vi "Autonomous Independent.vi"() -> ()   [LabVIEW 2015]
doc: "This VI is called when autonomous begins, and will automatically be terminated when autonomous ends. You can carry out timed or sensor driven robot movement independently without needing to return to the caller."
uses:
  <vilib>/Rock Robotics/WPI/Relay/WPI_RelayValue.ctl
  AutonEnum.ctl
  AutonEnumGoAround.ctl
  <vilib>/Rock Robotics/WPI/Utilities/WPI_GetSetVariantRefNum.vi
  Robot Values.vi
  DriveGlobal.vi
  <vilib>/Rock Robotics/WPI/RobotDrive/WPI_RobotDriveArcadeDrive_Standard(NoSaturation).vi
  Auton1ToteEnum.ctl
panel:
  in  "turn output range 5":cluster{"output high":dbl, "output low":dbl}={"output high"=0.8, "output low"=-0.8} {"output low" format="%.2f"; "output high" format="%.2f"}
  in  "PID Turn  gains 5":T1={"proportional gain (Kc)"=0.20000000000000004, "integral time (Ti, min)"=0.0, "derivative time (Td, min)"=0.0} {"derivative time (Td, min)" format="%.3f"; "integral time (Ti, min)" format="%.3f"; "proportional gain (Kc)" format="%.3f"}
  out "Total totes 4":i32
  in  "PID Turn  gains 4":T1={"proportional gain (Kc)"=0.20000000000000004, "integral time (Ti, min)"=0.0, "derivative time (Td, min)"=0.0} {"derivative time (Td, min)" format="%.3f"; "integral time (Ti, min)" format="%.3f"; "proportional gain (Kc)" format="%.3f"}
  in  "turn output range 4":cluster{"output high":dbl, "output low":dbl}={"output high"=0.8000000000000003, "output low"=-0.8000000000000002} {"output low" format="%.2f"; "output high" format="%.2f"}
  out "Total totes 3":i32
  in  "PID Turn  gains 3":T1={"proportional gain (Kc)"=0.05, "integral time (Ti, min)"=0.01, "derivative time (Td, min)"=0.0} {"derivative time (Td, min)" format="%.3f"; "integral time (Ti, min)" format="%.3f"; "proportional gain (Kc)" format="%.3f"}
  in  "turn output range 3":cluster{"output high":dbl, "output low":dbl}={"output high"=0.4, "output low"=-0.4} {"output low" format="%.2f"; "output high" format="%.2f"}
  out "Total totes 2":i32
  in  "PID Turn  gains 2":T1={"proportional gain (Kc)"=0.05, "integral time (Ti, min)"=0.01, "derivative time (Td, min)"=0.0} {"derivative time (Td, min)" format="%.3f"; "integral time (Ti, min)" format="%.3f"; "proportional gain (Kc)" format="%.3f"}
  in  "turn output range 2":cluster{"output high":dbl, "output low":dbl}={"output high"=0.4, "output low"=-0.4} {"output low" format="%.2f"; "output high" format="%.2f"}
  in  "Average gains 2":T1={"proportional gain (Kc)"=0.05, "integral time (Ti, min)"=0.0, "derivative time (Td, min)"=0.0}
  in  "output range":cluster{"output high":dbl, "output low":dbl}={"output high"=0.85, "output low"=-0.85}
  out "Total totes":i32
  out "Totes grabed":i32
  in  "PID Turn  gains":T1={"proportional gain (Kc)"=0.09999999999999999, "integral time (Ti, min)"=0.01, "derivative time (Td, min)"=0.0} {"derivative time (Td, min)" format="%.3f"; "integral time (Ti, min)" format="%.3f"; "proportional gain (Kc)" format="%.3f"}
  in  "turn output range":cluster{"output high":dbl, "output low":dbl}={"output high"=0.7, "output low"=-0.7} {"output low" format="%.2f"; "output high" format="%.2f"}
  in  "Average gains":T1={"proportional gain (Kc)"=0.01, "integral time (Ti, min)"=0.0, "derivative time (Td, min)"=0.0} {"derivative time (Td, min)" format="%.3f"; "integral time (Ti, min)" format="%.4f"; "proportional gain (Kc)" format="%.3f"}
  in  "name or relative path":string
  in  "P2":dbl[][](array[numeric])
  in  "P1":dbl[][](array[numeric])
  out "Current Movement, for debugging":T2 {"Y Joystick Value" scale=1.0..-1.0; "X Joystick Value" scale=-1.0..1.0}
  in  "Array of robot movements":T3(array[cluster]) {"Y Joystick Value" scale=1.0..-1.0; "X Joystick Value" scale=-1.0..1.0}
  # "Be sure to right-click and choose Data Operations>>Make Current Value default if you want to save the array values with the VI"
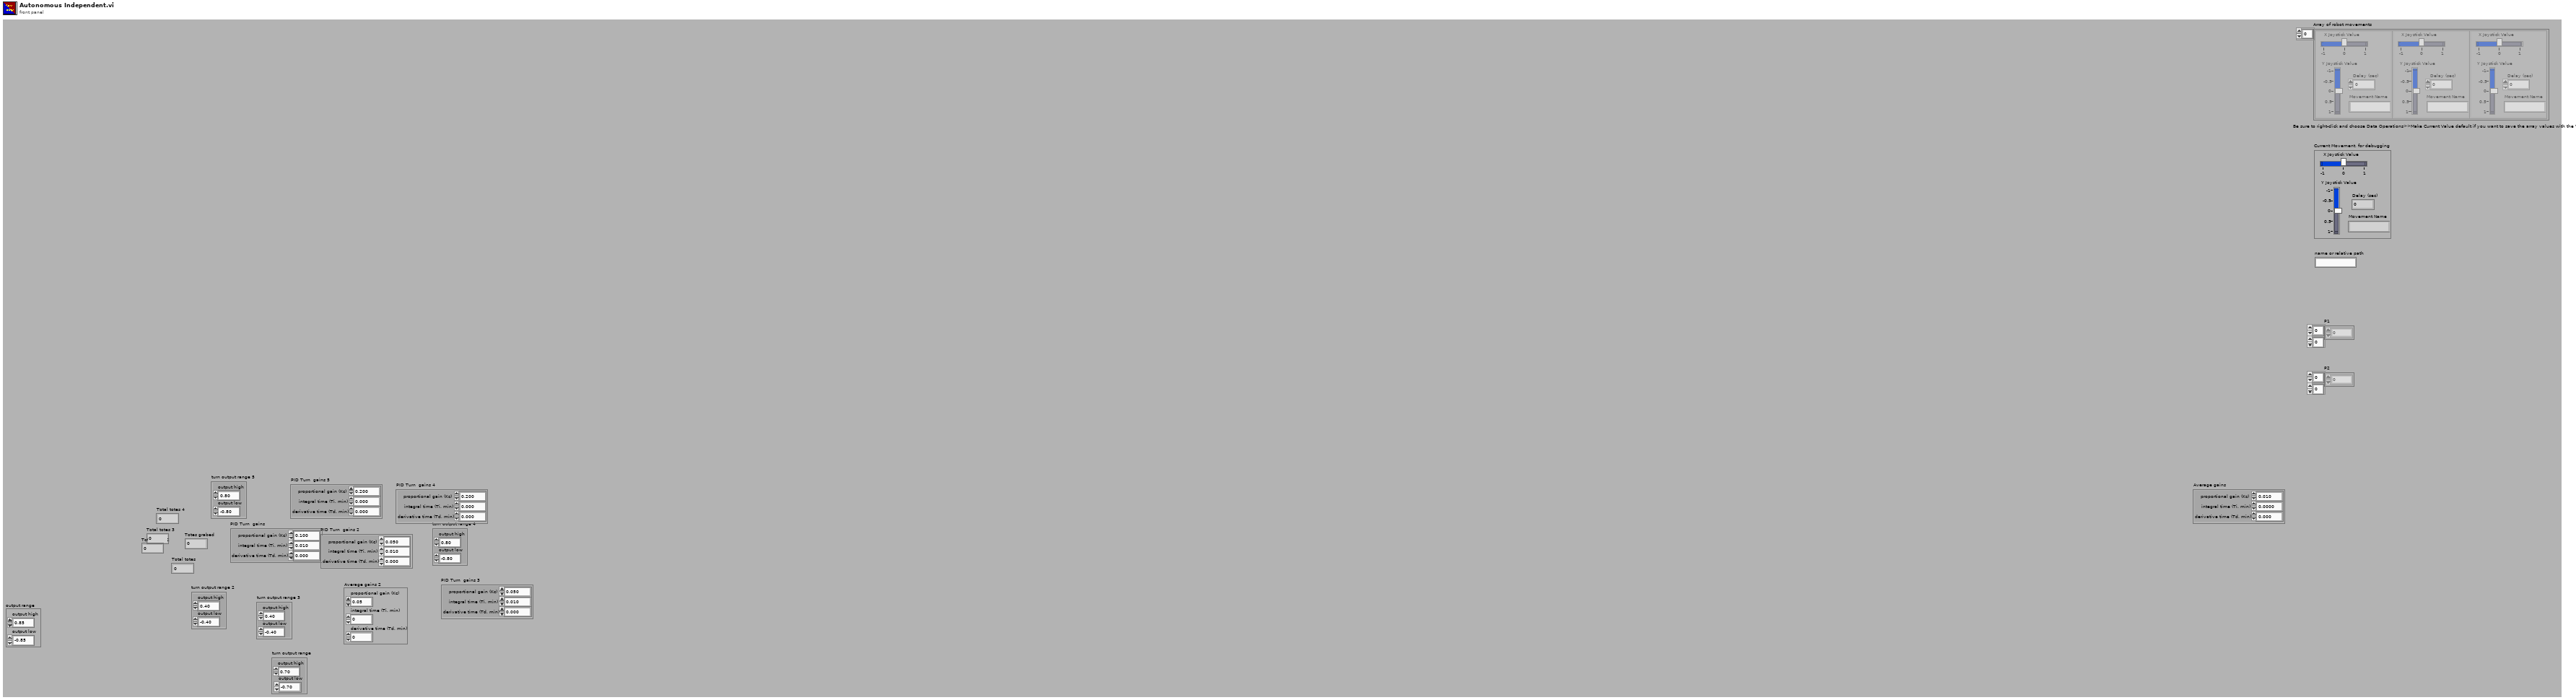
[diagram p1: front panel]
types:
  T1 = cluster{"proportional gain (Kc)":dbl, "integral time (Ti, min)":dbl, "derivative time (Td, min)":dbl}
  T2 = cluster{"X Joystick Value":dbl, "Y Joystick Value":dbl, "Delay (sec)":dbl, "Movement Name":string}
  T3 = cluster{"X Joystick Value":dbl, "Y Joystick Value":dbl, "Delay (sec)":dbl, "Movement Name":string}[]
  T4 = enum16{"Nothing", "Start", "Push", "Finish", "Turn", "Stack"}
  T5 = typedef "WPI_RelayValue.ctl" = enum16{"Off", "On", "Forward", "Reverse"}
  T6 = enum16{"Nothing", "Start", "Push", "Finish", "Turn", "Stack", "Back up"}
  T7 = typedef "AutonEnum.ctl" = enum16{"Go Around", "Nothing", "Start", "Push", "Release Totes", "Turn", "To Auto", "Stack", "Finish"}
  T8 = typedef "AutonEnumGoAround.ctl" = enum16{"Turn Right 1", "Go Straight 1", "Turn Left 1", "Go Straight 2", "Turn Left 2", "Go Straight 3", "Turn Right 3", "Go Straight 4", "Nothing"}
  T9 = typedef "Auton1ToteEnum.ctl" = enum16{"Start", "First Forward", "Get First Tote", "First Pick Up", "Stop"}
  T10 = cluster{"RightMotorSpeed":dbl, "LeftMotorSpeed":dbl}
  T11 = cluster{"Tracking Tote?":bool, "ToteRightSpeed":dbl, "ToteLeftSpeed":dbl, "Drive Encoder reset":bool, "Right Wheel \n(Cm)":dbl, "Left Wheel \n(Cm)":dbl}
  T12 = cluster{"Lift Position":i32, "Lift Speed Override":dbl, "OverrideTele?":bool, "OverrideDash":bool}
  T13 = cluster{"Lift Encoder Height Right (cm)":dbl, "Lift Encoder Height Left (cm)":dbl, "Right Prox":bool, "Left Prox":bool, "Gyro Angle":dbl, "Gyro anglar rate":dbl, "Gyro Reset":bool, "Drive encoder Dash reset":bool}
  T14 = typedef "WPI_JoystickDevRef.ctl" = cluster{"Device":T15}
  T15 = typedef "WPI_JoystickDeviceEnum.ctl" = enum16{"USB 0", "USB 1", "USB 2", "USB 3", "USB 4", "USB 5"}
  T16 = typedef "WPI_RobotDriveDevRef.ctl" = cluster{"DevStatus":errorcluster, "Motors[]":T17[], "Square Inputs":bool, "Max Output":dbl}
  T17 = typedef "WPI_MotorControlDeviceRef.ctl" = cluster{"DeviceStatus":errorcluster, "Type":T18, "PWM":cluster{"PWM Channel":T19, "DeadBand":T20}, "CAN":cluster{"Device Number":u8, "Control Mode":T21, "Semaphore":T22, "Max Vout":dbl, "TalonSRX Control Mode":T23}, "Invert":bool}
  T18 = typedef "WPI_MotorControlType.ctl" = enum16{"PWM", "CAN", "CANTalonSRX"}
  T19 = typedef "FPGA_DIOPWMChannel.ctl" = enum8{"PWM 0", "PWM 1", "PWM 2", "PWM 3", "PWM 4", "PWM 5", "PWM 6", "PWM 7", "PWM 8", "PWM 9", "PWM MXP 0", "PWM MXP 1", "PWM MXP 2", "PWM MXP 3", "PWM MXP 4", "PWM MXP 5", "PWM MXP 6", "PWM MXP 7", "PWM MXP 8", "PWM MXP 9", "Invalid"}
  T20 = typedef "WPI_PWMDeadband.ctl" = cluster{"Name":string, "maxPositivePwm":i32, "minPositivePwm":i32, "centerPwm":i32, "maxNegativePwm":i32, "minNegativePwm":i32, "angularRange":u16}
  T21 = typedef "WPI_CANJaguar_ControlMode.ctl" = enum8{"Percent VBus", "Current", "Speed", "Position", "Voltage"}
  T22 = typedef "Semaphore RefNum" = refnum<k1>
  T23 = typedef "WPI_CANTalonSRX_APIControlMode.ctl" = enum8{"Percent VBus", "Speed", "Position", "Slave", "Unchanged / Invalid", "Voltage Compensation", "Current", "Motion Profile"}
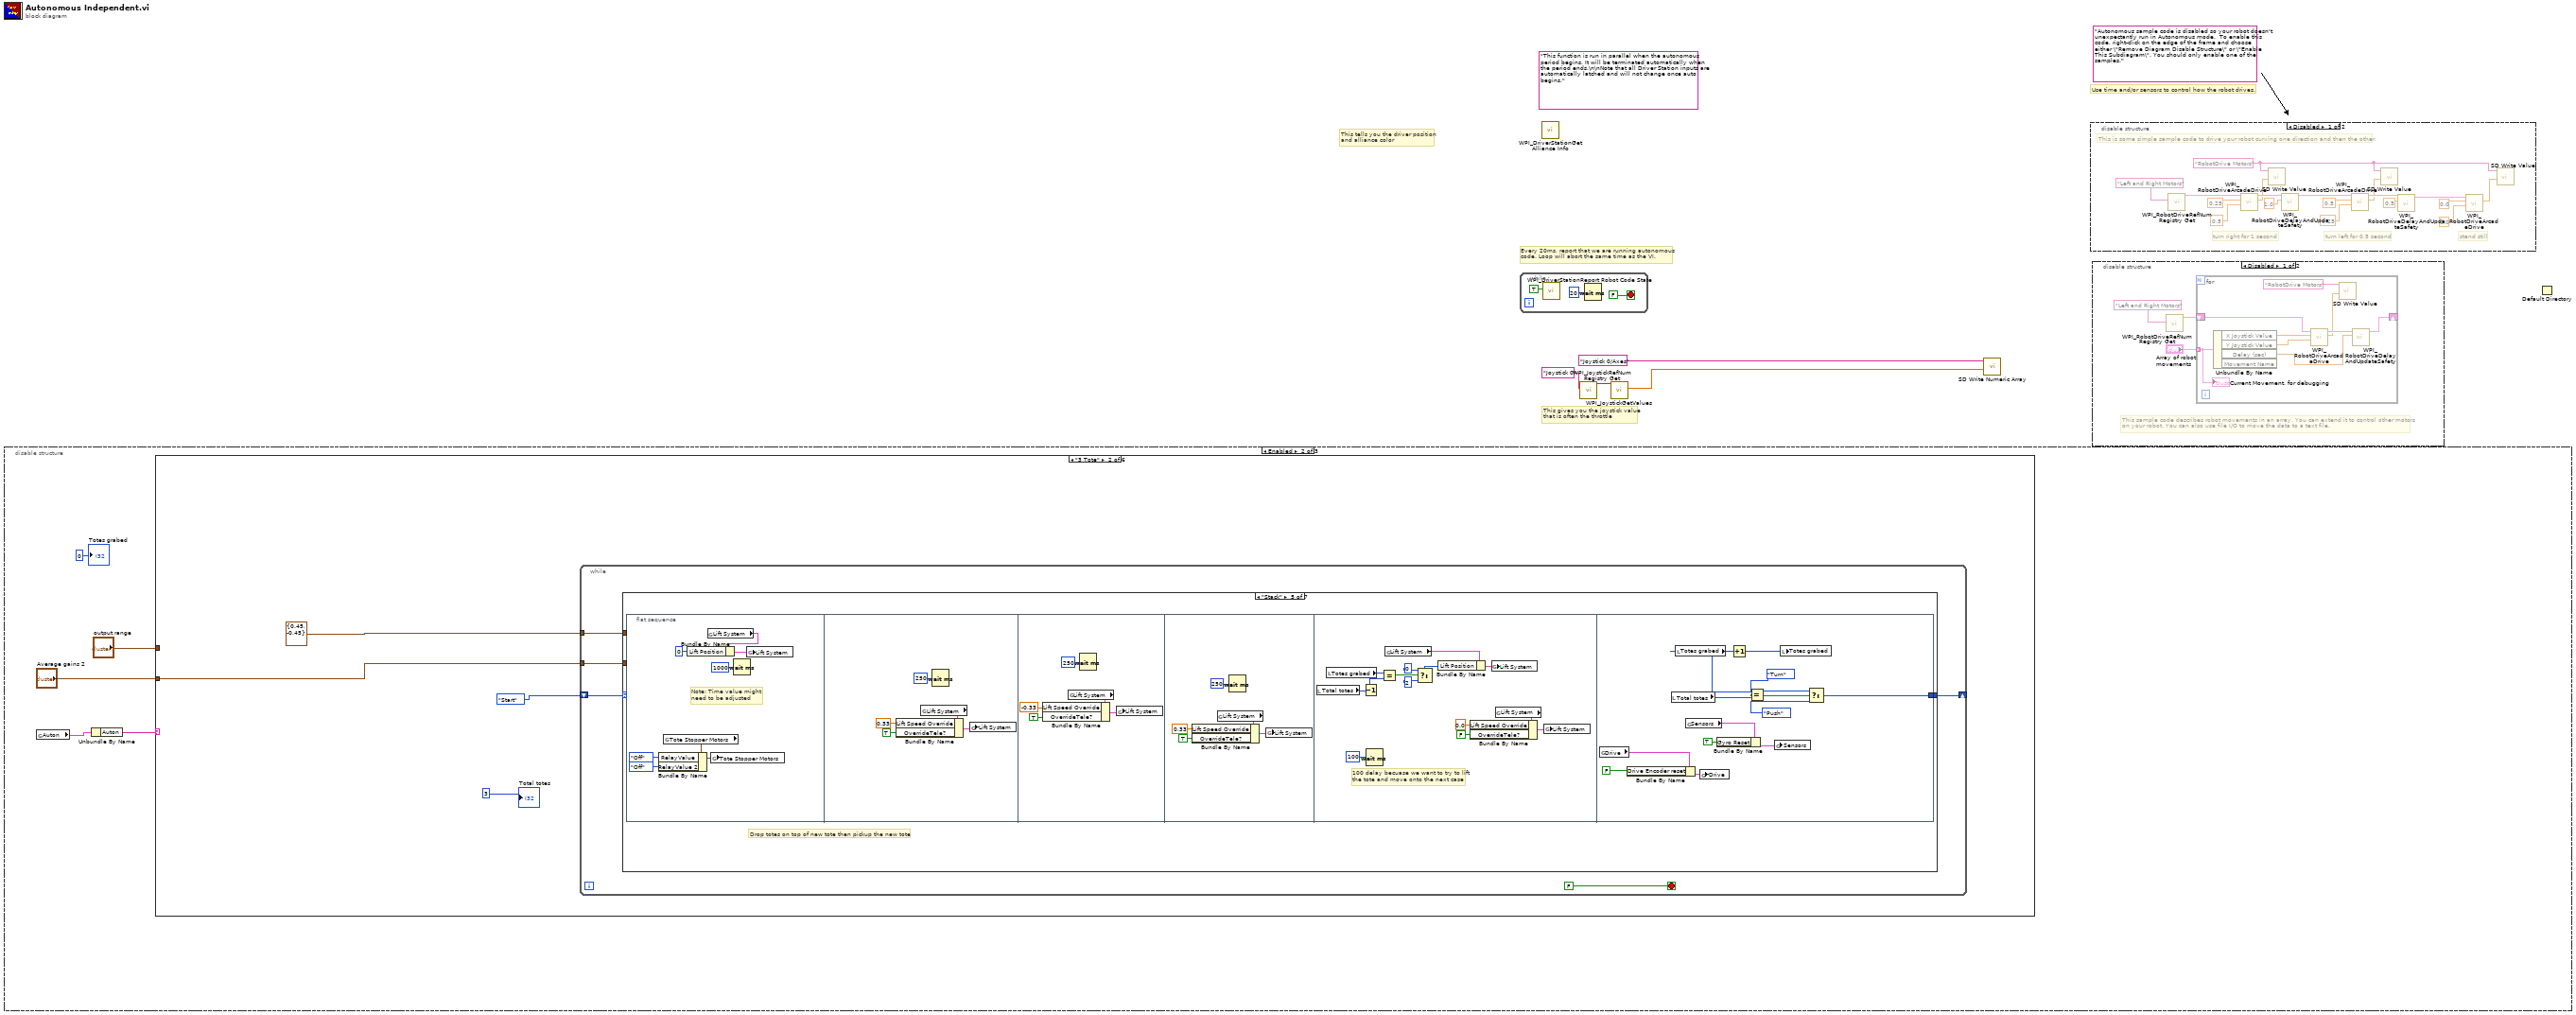
[diagram p0: block diagram]
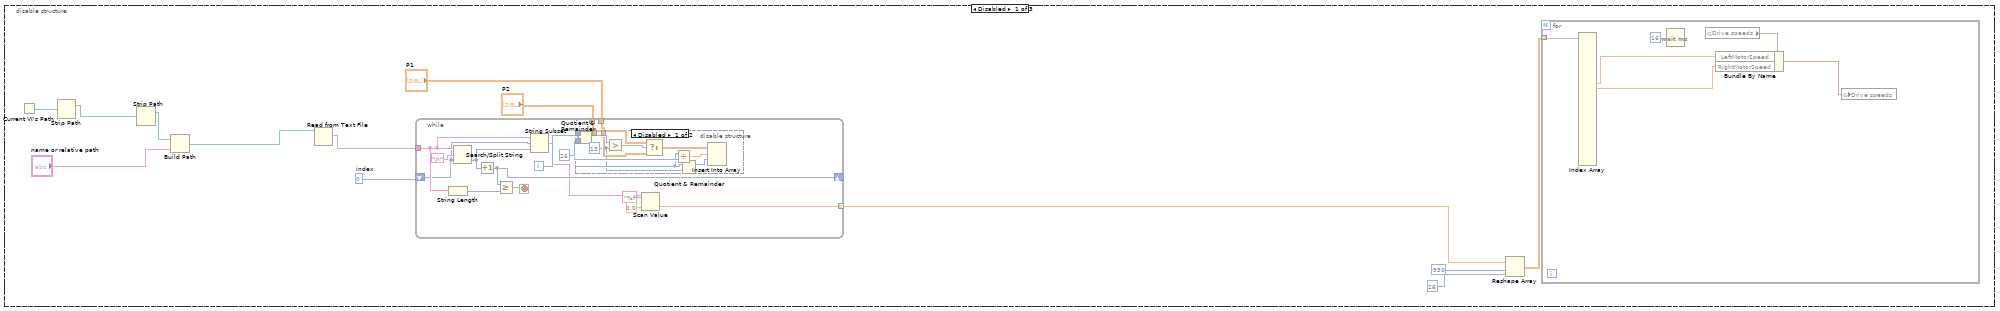
[diagram p2: hidden frame]
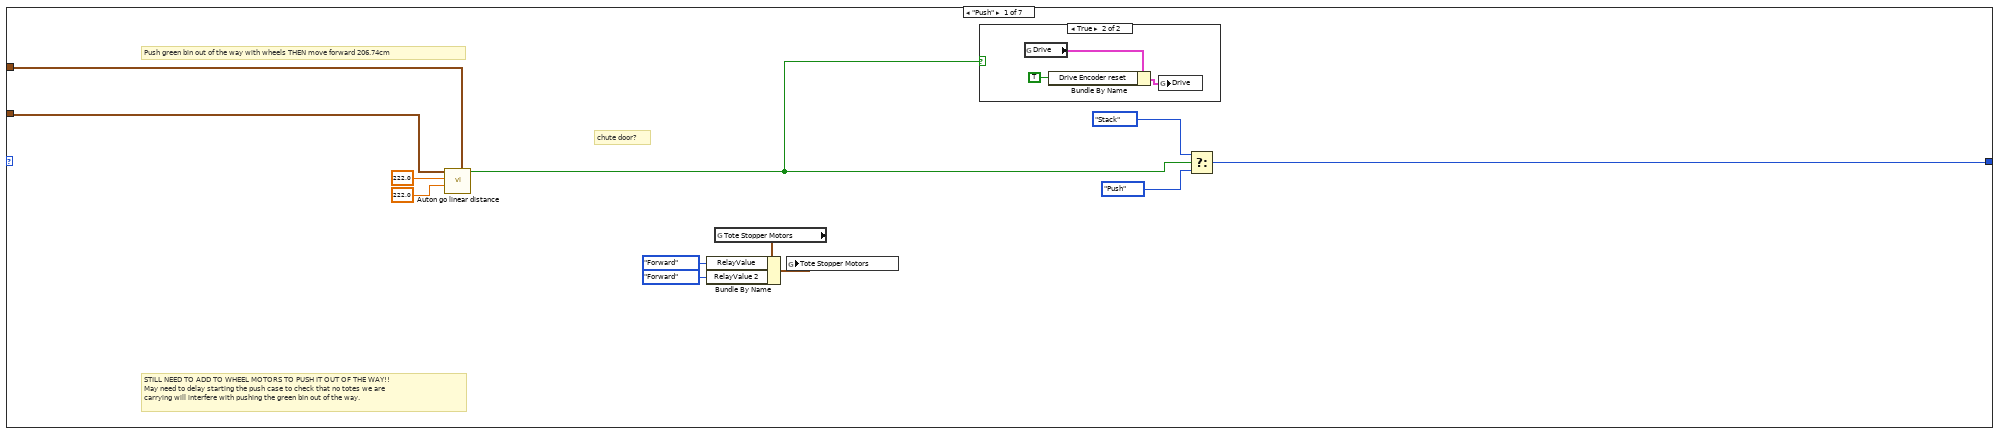
[diagram p5: hidden frame]
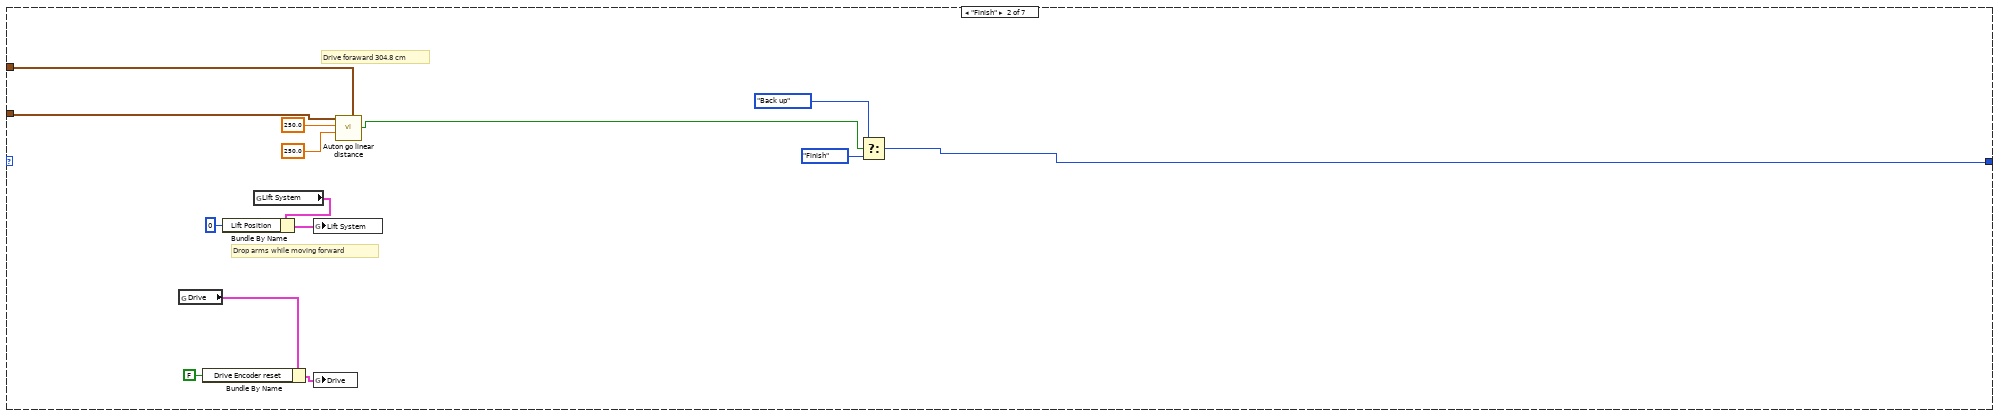
[diagram p7: hidden frame]
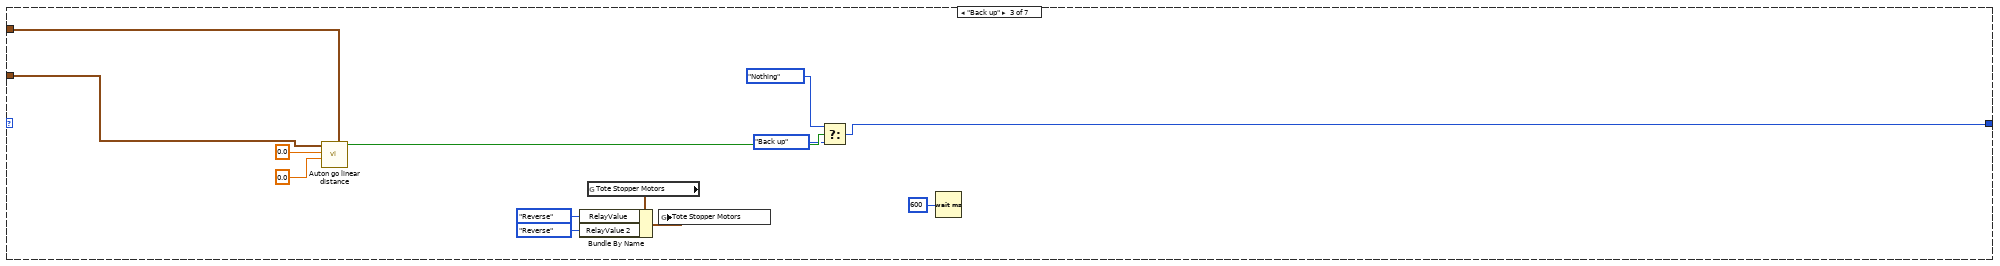
[diagram p8: hidden frame]
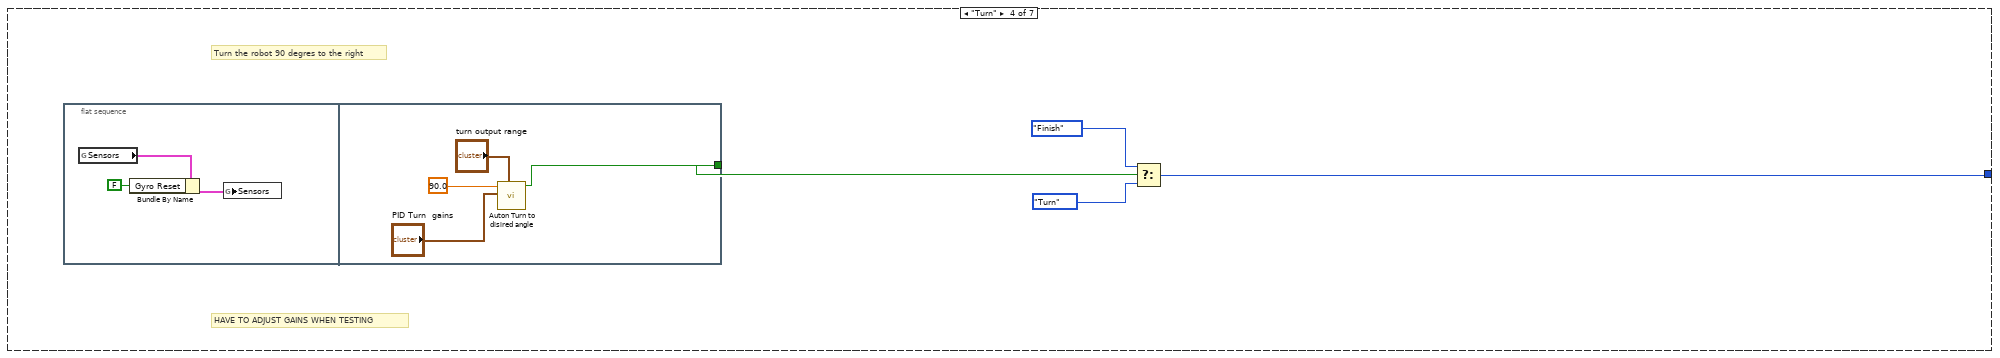
[diagram p9: hidden frame]
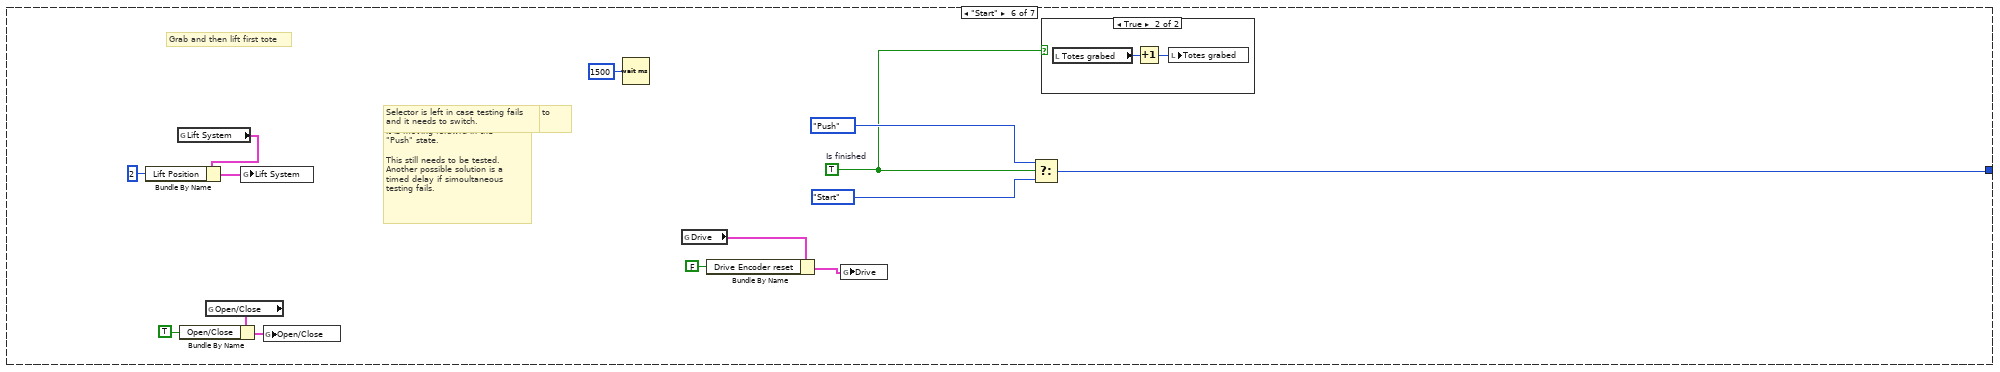
[diagram p10: hidden frame]
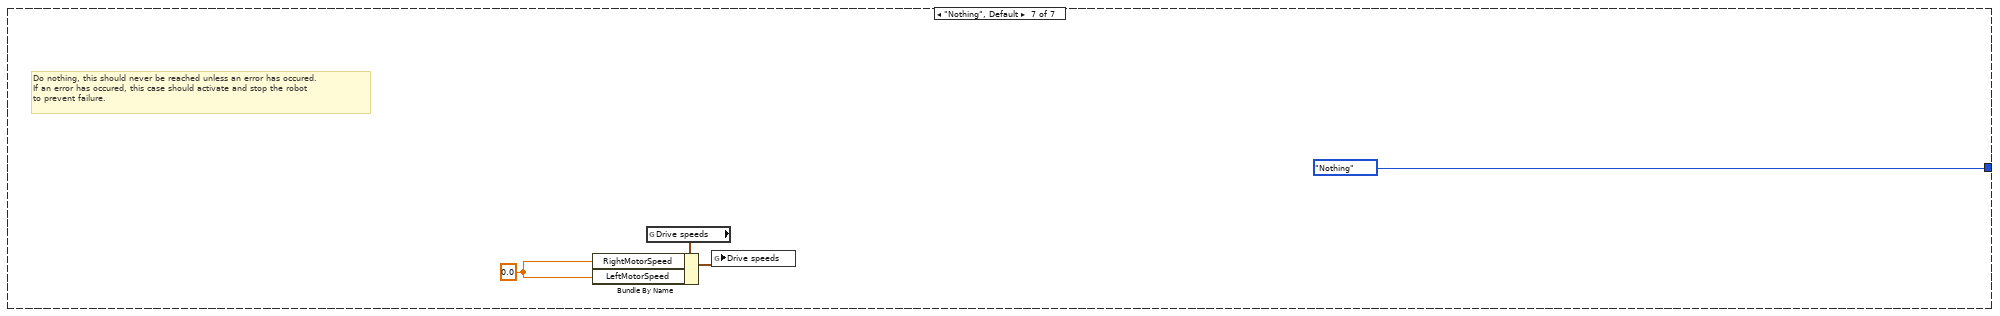
[diagram p12: hidden frame]
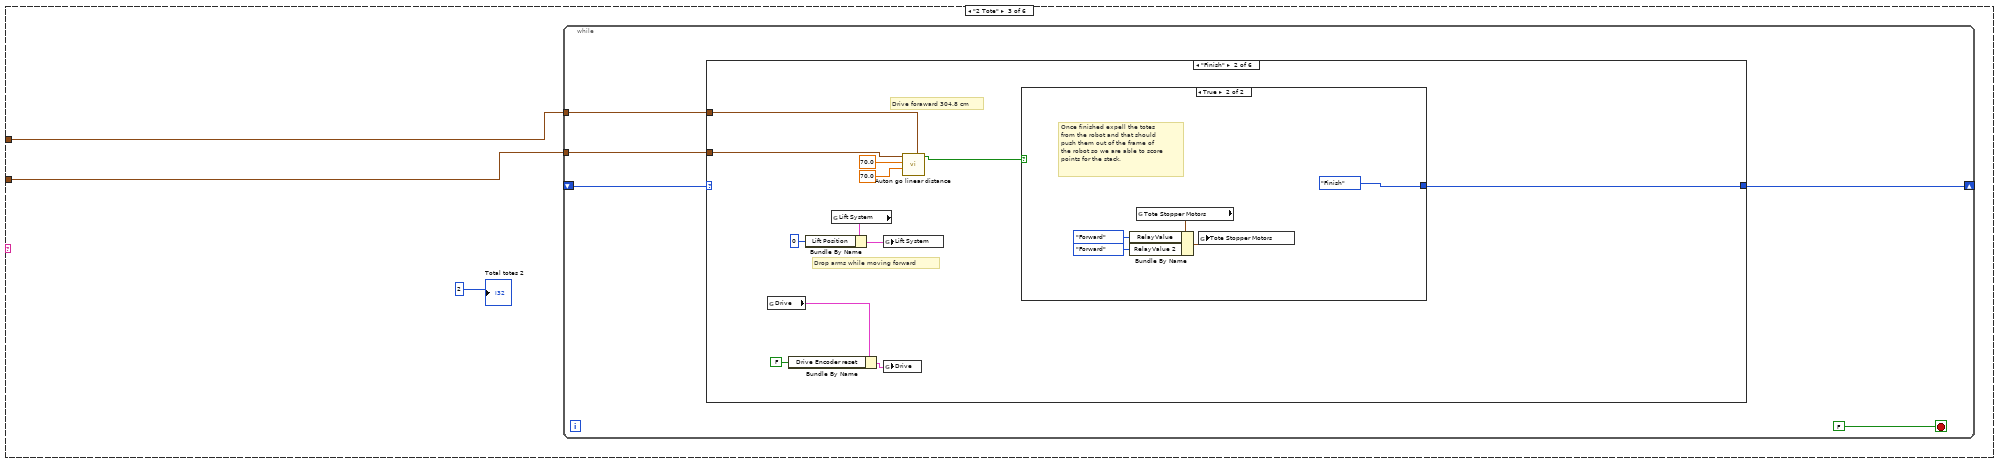
[diagram p13: hidden frame]
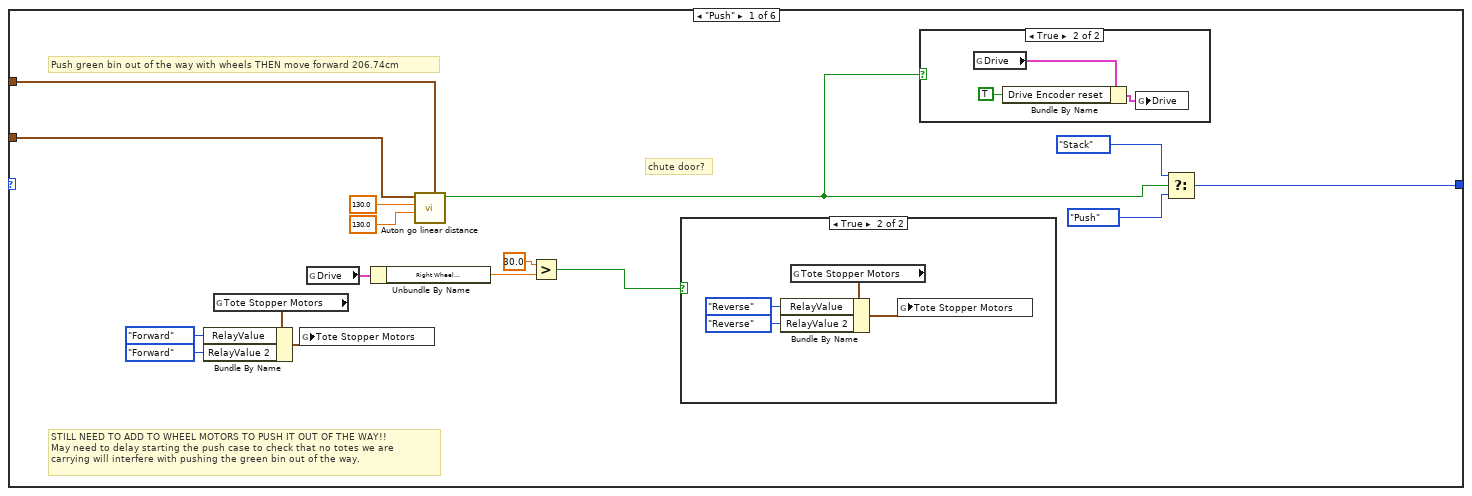
[diagram p14: hidden frame]
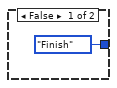
[diagram p17: hidden frame]
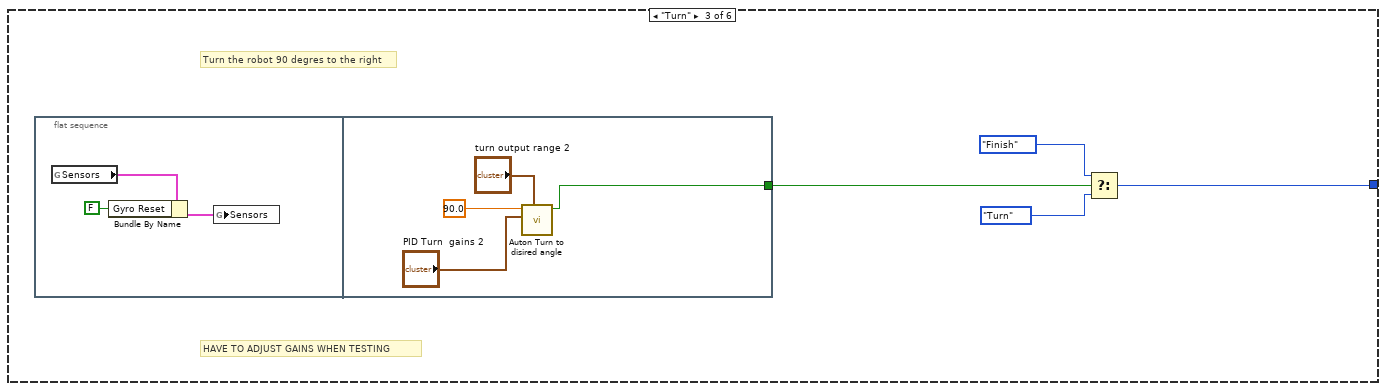
[diagram p18: hidden frame]
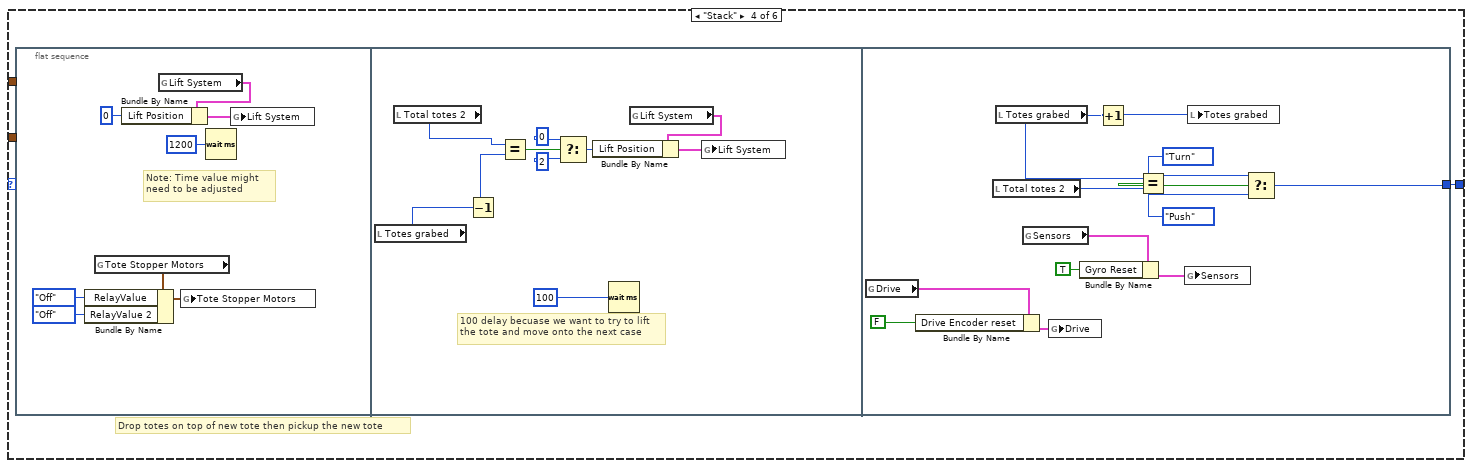
[diagram p19: hidden frame]
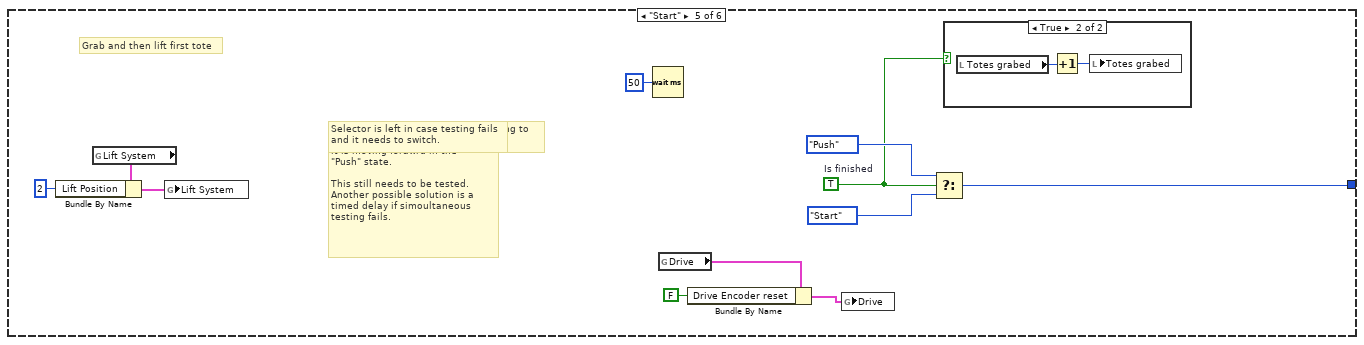
[diagram p20: hidden frame]
diagram:
  (unwired) "Autonomous sample code is disabled so your robot doesn't unexpectantly run in Autonomous mode.  To enable this code, right-click on the edge of the frame and choose either \"Remove Diagram Disable Structure\" or \"Enable This Subdiagram\". You should only enable one of the samples."
  (unwired) "This function is run in parallel when the autonomous period begins. It will be terminated automatically when the period ends.\n\nNote that all Driver Station inputs are automatically latched and will not change once auto begins."
  # "Every 20ms, report that we are running autonomous\ncode. Loop will abort the same time as the VI."
  # "This gives you the joystick value\nthat is often the throttle"
  # "Use time and/or sensors to control how the robot drives."
  # "This tells you the driver position\nand alliance color"
  n1 = disable-structure shown="Enabled" {
    frame Disabled {
      w16 = 0  # index
      n2 = Current VI's Path() -> (path=w10:path)
      n3 = Strip Path(path=w10) -> (stripped path=w9:path)  [unwired: 1 out]
      n4 = Strip Path(path=w9) -> (stripped path=w8:path)  [unwired: 1 out]
      n5 = Build Path(base path=w8, name or relative path="name or relative path") -> (appended path=w7:path)
      n6 = Read from Text File(file (use dialog)=w7) -> (text=w17:string)  [unwired: 3 in, 3 out]
      n7 = while {
        tunnel: w17 -> [w34]
        shift-right: [w35] -> _
        shift-left: w16 -> [w33]
        tunnel: "P1" -> [w30]
        tunnel: "P2" -> [w31]
        tunnel: [w27] -> w13 mode=indexing
        i -> [w28]
        stop <- w37 stop-if-true
        n8 = String Length(string=w34) -> (length=w38:i32)
        n9 = Search/Split String(string=w34, search string/char (-)="\n", offset (0)=w33) -> (offset of match=w32:i32)  [unwired: 2 out]
        n10 = Increment(x=w32) -> (x+1=w35:i32)
        n11 = Greater Or Equal?(x=w35, y=w38) -> (x >= y?=w37:bool)
        n12 = String Subset(string=w34, offset (0)=w33, length (rest)=w32) -> (substring=w26:string)
        n13 = disable-structure shown="Disabled" {
          disable-tunnel: w31 -> [w46 _]
          disable-tunnel: w30 -> [w45 _]
          disable-tunnel: 26 ("y") -> [w42 _]
          disable-tunnel: w28 -> [w40 _]
          frame Disabled {
            w39 = 13 ("y")
            n14 = Quotient & Remainder(x=w40, y=w42) -> (x-y*floor(x/y)=w48:i32)  [unwired: 1 out]
            n15 = Greater?(x=w48, y=w39) -> (0:w47:bool)
            n16 = Select(t=w46, s=w47, f=w45) -> (s? t:f=w44:dbl[][])
            n17 = Divide(x=w40, y=w42) -> (x/y=w43:dbl)
            n18 = Quotient & Remainder(x=w40, y=w39) -> (x-y*floor(x/y)=w41:i32)  [unwired: 1 out]
            n19 = Insert Into Array(array=w44, index (row)=w43, index (col)=w41) -> ()  [unwired: 1 in, 1 out]
          }
          frame Enabled {
          }
        }
        n20 = Scan Value(string=w26, format string="%f", default (0 dbl)=0.0 ("default (0 I32)")) -> (value=w27:dbl)  [unwired: 1 out]
      }
      n21 = Reshape Array(w13, 950 ("dimension size"), 26 ("dimension size")) -> (w5:dbl[][])
      n22 = for {
        tunnel: w5 -> [w23] mode=indexing
        n23 = Index Array(array=w23) -> (element #9=w21:dbl, element #10=w20:dbl)  [unwired: 26 in, 24 out]
        n24 = Wait (ms)(milliseconds to wait=u32 16) -> ()  [unwired: 1 out]
        n25 = global read "DriveGlobal.vi" "Drive speeds"() -> (w19:T10)
        n26 = Bundle By Name(cluster=w19, "LeftMotorSpeed"=w21, "RightMotorSpeed"=w20) -> (w18:T10)
        n27 = global write "DriveGlobal.vi" "Drive speeds"(w18) -> ()
      }
    }
    frame Enabled {
      n28 = global read "Robot Values.vi" "Auton"() -> (w50:cluster{"Auton":string, "Pushing tote":bool})
      n29 = Unbundle By Name(w50) -> ("Auton"=w49:string)
      n30 = case shown="\"3 Tote\"" w49 {
        tunnel: "Average gains 2" -> [_ w54 w187 w294 w405 w430]
        tunnel: "output range" -> [_ _ w188 w293 _ w431]
        frame "False", Default {
        }
        frame "3 Tote" {
          n31 = while {
            shift-right: [w61] -> _
            shift-left: T4."Start" -> [w62]
            tunnel: w54 -> [w59]
            tunnel: cluster{"output high":dbl, "output low":dbl} {"output high"=0.45, "output low"=-0.45} ("output range") -> [w58]
            stop <- FALSE stop-if-true
            n32 = case shown="\"Stack\"" w62 {
              tunnel: [w72 w78 w92 w106 w116 w178 T4."Nothing"] -> w61
              tunnel: w59 -> [w70 w88 w97 _ _ _ _]
              tunnel: w58 -> [w71 w89 w96 _ _ _ _]
              frame "Push" {
                # "chute door?"
                # "STILL NEED TO ADD TO WHEEL MOTORS TO PUSH IT OUT OF THE WAY!!\nMay need to delay starting the push case to check that no totes we are \ncarrying will interfere with pushing the green bin out of the way."
                # "Push green bin out of the way with wheels THEN move forward 206.74cm"
                n33 = call "Auton go linear distance.vi"("Average gains"=w70, "PID setpoint"=222.0, "Goal"=222.0, "output range"=w71) -> ("Done?"=w68:bool)  [unwired: 4 in]
                n34 = global read "Robot Values.vi" "Tote Stopper Motors"() -> (w64:cluster{"RelayValue":T5, "RelayValue 2":T5})
                n35 = Bundle By Name(cluster=w64, "RelayValue"=WPI_RelayValue."Forward", "RelayValue 2"=WPI_RelayValue."Forward") -> (w63:cluster{"RelayValue":T5, "RelayValue 2":T5})
                n36 = global write "Robot Values.vi" "Tote Stopper Motors"(w63) -> ()
                n37 = case shown="True" w68 {
                  frame False {
                  }
                  frame True {
                    n38 = global read "Robot Values.vi" "Drive"() -> (w76:T11)
                    n39 = Bundle By Name(cluster=w76, "Drive Encoder reset"=TRUE) -> (w77:T11)
                    n40 = global write "Robot Values.vi" "Drive"(w77) -> ()
                  }
                }
                n41 = Select(t=T4."Stack", s=w68, f=T4."Push") -> (s? t:f=w72:T4)
              }
              frame "Finish" {
                # "Drop arms while moving forward"
                # "Drive foraward 304.8 cm"
                n42 = global read "Robot Values.vi" "Drive"() -> (w86:T11)
                n43 = Bundle By Name(cluster=w86, "Drive Encoder reset"=FALSE) -> (w87:T11)
                n44 = global read "Robot Values.vi" "Lift System"() -> (w83:T12)
                n45 = Bundle By Name(cluster=w83, "Lift Position"=0) -> (w84:T12)
                n46 = global write "Robot Values.vi" "Lift System"(w84) -> ()
                n47 = global write "Robot Values.vi" "Drive"(w87) -> ()
                n48 = call "Auton go linear distance.vi"("Average gains"=w88, "PID setpoint"=250.0, "Goal"=250.0, "output range"=w89) -> ("Done?"=w81:bool)  [unwired: 4 in]
                n49 = Select(t=T6."Back up", s=w81, f=T6."Finish") -> (s? t:f=w78:T6)
              }
              frame "Back up" {
                n50 = call "Auton go linear distance.vi"("Average gains"=w97, "PID setpoint"=0.0, "Goal"=0.0, "output range"=w96) -> ("Done?"=w95:bool)  [unwired: 4 in]
                n51 = global read "Robot Values.vi" "Tote Stopper Motors"() -> (w103:cluster{"RelayValue":T5, "RelayValue 2":T5})
                n52 = Bundle By Name(cluster=w103, "RelayValue"=WPI_RelayValue."Reverse", "RelayValue 2"=WPI_RelayValue."Reverse") -> (w104:cluster{"RelayValue":T5, "RelayValue 2":T5})
                n53 = global write "Robot Values.vi" "Tote Stopper Motors"(w104) -> ()
                n54 = Select(t=T6."Nothing", s=w95, f=T6."Back up") -> (s? t:f=w92:T6)
                n55 = Wait (ms)(milliseconds to wait=u32 600) -> ()  [unwired: 1 out]
              }
              frame "Turn" {
                # "HAVE TO ADJUST GAINS WHEN TESTING"
                # "Turn the robot 90 degres to the right"
                n56 = flat-sequence {
                  tunnel: [w112] -> w105
                  frame #0 {
                    n57 = global read "Robot Values.vi" "Sensors"() -> (w110:T13)
                    n58 = Bundle By Name(cluster=w110, "Gyro Reset"=FALSE) -> (w109:T13)
                    n59 = global write "Robot Values.vi" "Sensors"(w109) -> ()
                  }
                  frame #1 {
                    n60 = call "Auton Turn to disired angle.vi"("Power output range"="turn output range", "PID Turn  gains"="PID Turn  gains", "Angle setpoint"=90.0) -> ("In Range?"=w112:bool)  [unwired: 8 in]
                  }
                }
                n61 = Select(t=T4."Finish", s=w105, f=T4."Turn") -> (s? t:f=w106:T4)
              }
              frame "Stack" {
                # "Drop totes on top of new tote then pickup the new tote"
                n62 = flat-sequence {
                  tunnel: [w166] -> w116
                  frame #0 {
                    # "Note: Time value might \nneed to be adjusted"
                    n63 = global read "Robot Values.vi" "Tote Stopper Motors"() -> (w119:cluster{"RelayValue":T5, "RelayValue 2":T5})
                    n64 = Bundle By Name(cluster=w119, "RelayValue"=WPI_RelayValue."Off", "RelayValue 2"=WPI_RelayValue."Off") -> (w120:cluster{"RelayValue":T5, "RelayValue 2":T5})
                    n65 = global read "Robot Values.vi" "Lift System"() -> (w123:T12)
                    n66 = Bundle By Name(cluster=w123, "Lift Position"=0) -> (w122:T12)
                    n67 = global write "Robot Values.vi" "Tote Stopper Motors"(w120) -> ()
                    n68 = Wait (ms)(milliseconds to wait=u32 1000) -> ()  [unwired: 1 out]
                    n69 = global write "Robot Values.vi" "Lift System"(w122) -> ()
                  }
                  frame #1 {
                    n70 = global read "Robot Values.vi" "Lift System"() -> (w128:T12)
                    n71 = Bundle By Name(cluster=w128, "Lift Speed Override"=0.33, "OverrideTele?"=TRUE) -> (w129:T12)
                    n72 = Wait (ms)(milliseconds to wait=u32 250) -> ()  [unwired: 1 out]
                    n73 = global write "Robot Values.vi" "Lift System"(w129) -> ()
                  }
                  frame #2 {
                    n74 = global read "Robot Values.vi" "Lift System"() -> (w133:T12)
                    n75 = Bundle By Name(cluster=w133, "Lift Speed Override"=-0.33, "OverrideTele?"=TRUE) -> (w134:T12)
                    n76 = Wait (ms)(milliseconds to wait=u32 250) -> ()  [unwired: 1 out]
                    n77 = global write "Robot Values.vi" "Lift System"(w134) -> ()
                  }
                  frame #3 {
                    n78 = global read "Robot Values.vi" "Lift System"() -> (w138:T12)
                    n79 = Bundle By Name(cluster=w138, "Lift Speed Override"=0.33, "OverrideTele?"=TRUE) -> (w139:T12)
                    n80 = Wait (ms)(milliseconds to wait=u32 250) -> ()  [unwired: 1 out]
                    n81 = global write "Robot Values.vi" "Lift System"(w139) -> ()
                  }
                  frame #4 {
                    # "100 delay becuase we want to try to lift\nthe tote and move onto the next case"
                    n82 = local read "Total totes"() -> (w146:i32)
                    n83 = local read "Totes grabed"() -> (w144:i32)
                    n84 = Decrement(x=w146) -> (x-1=w145:i32)
                    n85 = Wait (ms)(milliseconds to wait=u32 100) -> ()  [unwired: 1 out]
                    n86 = Equal?(x=w144, y=w145) -> (x = y?=w150:bool)
                    n87 = global read "Robot Values.vi" "Lift System"() -> (w152:T12)
                    n88 = Select(t=0 ("Lift Position"), s=w150, f=2 ("Lift Position")) -> (s? t:f=w147:i32)
                    n89 = Bundle By Name(cluster=w152, "Lift Position"=w147) -> (w153:T12)
                    n90 = global write "Robot Values.vi" "Lift System"(w153) -> ()
                    n91 = global read "Robot Values.vi" "Lift System"() -> (w142:T12)
                    n92 = Bundle By Name(cluster=w142, "Lift Speed Override"=0.0, "OverrideTele?"=FALSE) -> (w143:T12)
                    n93 = global write "Robot Values.vi" "Lift System"(w143) -> ()
                  }
                  frame #5 {
                    n94 = global read "Robot Values.vi" "Drive"() -> (w155:T11)
                    n95 = Bundle By Name(cluster=w155, "Drive Encoder reset"=FALSE) -> (w156:T11)
                    n96 = local read "Total totes"() -> (w163:i32)
                    n97 = local read "Totes grabed"() -> (w165:i32)
                    n98 = global read "Robot Values.vi" "Sensors"() -> (w158:T13)
                    n99 = global write "Robot Values.vi" "Drive"(w156) -> ()
                    n100 = Bundle By Name(cluster=w158, "Gyro Reset"=TRUE) -> (w159:T13)
                    n101 = Increment(x=w165) -> (x+1=w164:i32)
                    n102 = Equal?(x=w164, y=w163) -> (x = y?=w161:bool)
                    n103 = global write "Robot Values.vi" "Sensors"(w159) -> ()
                    n104 = local write "Totes grabed"(w164) -> ()
                    n105 = Select(t=T4."Turn", s=w161, f=T4."Push") -> (s? t:f=w166:T4)
                  }
                }
              }
              frame "Start" {
                w177 = TRUE  # Is finished
                # "Selector is left in case testing fails\nand it needs to switch."
                # "Will switch to push state after starting to\nlift the tote."
                # "Is finished is set to true because\nthe robot will lift the tote while\nit is moving forawrd in the\n\"Push\" state.\n\nThis still needs to be tested.\nAnother possible solution is a\ntimed delay if simoultaneous\ntesting fails."
                # "Grab and then lift first tote"
                n106 = global read "Robot Values.vi" "Lift System"() -> (w175:T12)
                n107 = Bundle By Name(cluster=w175, "Lift Position"=2) -> (w176:T12)
                n108 = global read "Robot Values.vi" "Open/Close"() -> (w168:cluster{"Open/Close":bool})
                n109 = Bundle By Name(cluster=w168, "Open/Close"=TRUE) -> (w169:cluster{"Open/Close":bool})
                n110 = global write "Robot Values.vi" "Lift System"(w176) -> ()
                n111 = global write "Robot Values.vi" "Open/Close"(w169) -> ()
                n112 = Wait (ms)(milliseconds to wait=u32 1500) -> ()  [unwired: 1 out]
                n113 = global read "Robot Values.vi" "Drive"() -> (w172:T11)
                n114 = Bundle By Name(cluster=w172, "Drive Encoder reset"=FALSE) -> (w173:T11)
                n115 = global write "Robot Values.vi" "Drive"(w173) -> ()
                n116 = Select(t=T4."Push", s=w177, f=T4."Start") -> (s? t:f=w178:T4)
                n117 = case shown="True" w177 {
                  frame False {
                  }
                  frame True {
                    n118 = local read "Totes grabed"() -> (w182:i32)
                    n119 = Increment(x=w182) -> (x+1=w181:i32)
                    n120 = local write "Totes grabed"(w181) -> ()
                  }
                }
              }
              frame "Nothing", Default {
                w183 = 0.0
                # "Do nothing, this should never be reached unless an error has occured.\nIf an error has occured, this case should activate and stop the robot\nto prevent failure."
                n121 = global read "DriveGlobal.vi" "Drive speeds"() -> (w185:T10)
                n122 = Bundle By Name(cluster=w185, "RightMotorSpeed"=w183, "LeftMotorSpeed"=w183) -> (w184:T10)
                n123 = global write "DriveGlobal.vi" "Drive speeds"(w184) -> ()
              }
            }
          }
          "Total totes" <- 3 ("Total totes")
        }
        frame "2 Tote" {
          n124 = while {
            shift-right: [w193] -> _
            shift-left: _ -> [w194]
            tunnel: w187 -> [w191]
            tunnel: w188 -> [w190]
            stop <- FALSE stop-if-true
            n125 = case shown="\"Finish\"" w194 {
              tunnel: [w208 w221 w237 w247 w287 T4."Nothing"] -> w193
              tunnel: w191 -> [w206 w226 _ _ _ _]
              tunnel: w190 -> [w207 w227 _ _ _ _]
              frame "Push" {
                # "chute door?"
                # "STILL NEED TO ADD TO WHEEL MOTORS TO PUSH IT OUT OF THE WAY!!\nMay need to delay starting the push case to check that no totes we are \ncarrying will interfere with pushing the green bin out of the way."
                # "Push green bin out of the way with wheels THEN move forward 206.74cm"
                n126 = global read "Robot Values.vi" "Tote Stopper Motors"() -> (w203:cluster{"RelayValue":T5, "RelayValue 2":T5})
                n127 = Bundle By Name(cluster=w203, "RelayValue"=WPI_RelayValue."Forward", "RelayValue 2"=WPI_RelayValue."Forward") -> (w204:cluster{"RelayValue":T5, "RelayValue 2":T5})
                n128 = global write "Robot Values.vi" "Tote Stopper Motors"(w204) -> ()
                n129 = global read "Robot Values.vi" "Drive"() -> (w198:T11)
                n130 = Unbundle By Name(w198) -> ("Right Wheel \n(Cm)"=w196:dbl)
                n131 = call "Auton go linear distance.vi"("Average gains"=w206, "PID setpoint"=130.0, "Goal"=130.0, "output range"=w207) -> ("Done?"=w200:bool)  [unwired: 4 in]
                n132 = Greater?(x=30.0, y=w196) -> (0:w195:bool)
                n133 = case shown="True" w195 {
                  frame False {
                  }
                  frame True {
                    n134 = global read "Robot Values.vi" "Tote Stopper Motors"() -> (w212:cluster{"RelayValue":T5, "RelayValue 2":T5})
                    n135 = Bundle By Name(cluster=w212, "RelayValue"=WPI_RelayValue."Reverse", "RelayValue 2"=WPI_RelayValue."Reverse") -> (w211:cluster{"RelayValue":T5, "RelayValue 2":T5})
                    n136 = global write "Robot Values.vi" "Tote Stopper Motors"(w211) -> ()
                  }
                }
                n137 = case shown="True" w200 {
                  frame False {
                  }
                  frame True {
                    n138 = global read "Robot Values.vi" "Drive"() -> (w216:T11)
                    n139 = Bundle By Name(cluster=w216, "Drive Encoder reset"=TRUE) -> (w217:T11)
                    n140 = global write "Robot Values.vi" "Drive"(w217) -> ()
                  }
                }
                n141 = Select(t=T4."Stack", s=w200, f=T4."Push") -> (s? t:f=w208:T4)
              }
              frame "Finish" {
                # "Drop arms while moving forward"
                # "Drive foraward 304.8 cm"
                n142 = global read "Robot Values.vi" "Drive"() -> (w223:T11)
                n143 = Bundle By Name(cluster=w223, "Drive Encoder reset"=FALSE) -> (w224:T11)
                n144 = global read "Robot Values.vi" "Lift System"() -> (w219:T12)
                n145 = Bundle By Name(cluster=w219, "Lift Position"=0) -> (w220:T12)
                n146 = global write "Robot Values.vi" "Lift System"(w220) -> ()
                n147 = global write "Robot Values.vi" "Drive"(w224) -> ()
                n148 = call "Auton go linear distance.vi"("Average gains"=w226, "PID setpoint"=70.0, "Goal"=70.0, "output range"=w227) -> ("Done?"=w225:bool)  [unwired: 4 in]
                n149 = case shown="True" w225 {
                  tunnel: [T4."Finish" T4."Finish"] -> w221
                  frame False {
                  }
                  frame True {
                    # "Once finished expell the totes\nfrom the robot and that should\npush them out of the frame of\nthe robot so we are able to score\npoints for the stack."
                    n150 = global read "Robot Values.vi" "Tote Stopper Motors"() -> (w233:cluster{"RelayValue":T5, "RelayValue 2":T5})
                    n151 = Bundle By Name(cluster=w233, "RelayValue"=WPI_RelayValue."Forward", "RelayValue 2"=WPI_RelayValue."Forward") -> (w234:cluster{"RelayValue":T5, "RelayValue 2":T5})
                    n152 = global write "Robot Values.vi" "Tote Stopper Motors"(w234) -> ()
                  }
                }
              }
              frame "Turn" {
                # "HAVE TO ADJUST GAINS WHEN TESTING"
                # "Turn the robot 90 degres to the right"
                n153 = flat-sequence {
                  tunnel: [w243] -> w236
                  frame #0 {
                    n154 = global read "Robot Values.vi" "Sensors"() -> (w241:T13)
                    n155 = Bundle By Name(cluster=w241, "Gyro Reset"=FALSE) -> (w240:T13)
                    n156 = global write "Robot Values.vi" "Sensors"(w240) -> ()
                  }
                  frame #1 {
                    n157 = call "Auton Turn to disired angle.vi"("Power output range"="turn output range 2", "PID Turn  gains"="PID Turn  gains 2", "Angle setpoint"=90.0) -> ("In Range?"=w243:bool)  [unwired: 8 in]
                  }
                }
                n158 = Select(t=T4."Finish", s=w236, f=T4."Turn") -> (s? t:f=w237:T4)
              }
              frame "Stack" {
                # "Drop totes on top of new tote then pickup the new tote"
                n159 = flat-sequence {
                  tunnel: [w278] -> w247
                  frame #0 {
                    # "Note: Time value might \nneed to be adjusted"
                    n160 = global read "Robot Values.vi" "Tote Stopper Motors"() -> (w250:cluster{"RelayValue":T5, "RelayValue 2":T5})
                    n161 = Bundle By Name(cluster=w250, "RelayValue"=WPI_RelayValue."Off", "RelayValue 2"=WPI_RelayValue."Off") -> (w251:cluster{"RelayValue":T5, "RelayValue 2":T5})
                    n162 = global read "Robot Values.vi" "Lift System"() -> (w254:T12)
                    n163 = Bundle By Name(cluster=w254, "Lift Position"=0) -> (w253:T12)
                    n164 = global write "Robot Values.vi" "Tote Stopper Motors"(w251) -> ()
                    n165 = Wait (ms)(milliseconds to wait=u32 1200) -> ()  [unwired: 1 out]
                    n166 = global write "Robot Values.vi" "Lift System"(w253) -> ()
                  }
                  frame #1 {
                    # "100 delay becuase we want to try to lift\nthe tote and move onto the next case"
                    n167 = local read "Totes grabed"() -> (w257:i32)
                    n168 = local read "Total totes 2"() -> (w258:i32)
                    n169 = Decrement(x=w257) -> (x-1=w256:i32)
                    n170 = Equal?(x=w258, y=w256) -> (x = y?=w262:bool)
                    n171 = Select(t=0 ("Lift Position"), s=w262, f=2 ("Lift Position")) -> (s? t:f=w259:i32)
                    n172 = Wait (ms)(milliseconds to wait=u32 100) -> ()  [unwired: 1 out]
                    n173 = global read "Robot Values.vi" "Lift System"() -> (w264:T12)
                    n174 = Bundle By Name(cluster=w264, "Lift Position"=w259) -> (w265:T12)
                    n175 = global write "Robot Values.vi" "Lift System"(w265) -> ()
                  }
                  frame #2 {
                    n176 = global read "Robot Values.vi" "Drive"() -> (w269:T11)
                    n177 = Bundle By Name(cluster=w269, "Drive Encoder reset"=FALSE) -> (w270:T11)
                    n178 = local read "Total totes 2"() -> (w277:i32)
                    n179 = local read "Totes grabed"() -> (w266:i32)
                    n180 = global read "Robot Values.vi" "Sensors"() -> (w272:T13)
                    n181 = global write "Robot Values.vi" "Drive"(w270) -> ()
                    n182 = Bundle By Name(cluster=w272, "Gyro Reset"=TRUE) -> (w273:T13)
                    n183 = Increment(x=w266) -> (x+1=w267:i32)
                    n184 = Equal?(x=w266, y=w277) -> (x = y?=w275:bool)
                    n185 = global write "Robot Values.vi" "Sensors"(w273) -> ()
                    n186 = local write "Totes grabed"(w267) -> ()
                    n187 = Select(t=T4."Turn", s=w275, f=T4."Push") -> (s? t:f=w278:T4)
                  }
                }
              }
              frame "Start" {
                w286 = TRUE  # Is finished
                # "Selector is left in case testing fails\nand it needs to switch."
                # "Will switch to push state after starting to\nlift the tote."
                # "Is finished is set to true because\nthe robot will lift the tote while\nit is moving forawrd in the\n\"Push\" state.\n\nThis still needs to be tested.\nAnother possible solution is a\ntimed delay if simoultaneous\ntesting fails."
                # "Grab and then lift first tote"
                n188 = global read "Robot Values.vi" "Lift System"() -> (w284:T12)
                n189 = Bundle By Name(cluster=w284, "Lift Position"=2) -> (w285:T12)
                n190 = global write "Robot Values.vi" "Lift System"(w285) -> ()
                n191 = Wait (ms)(milliseconds to wait=u32 50) -> ()  [unwired: 1 out]
                n192 = global read "Robot Values.vi" "Drive"() -> (w281:T11)
                n193 = Bundle By Name(cluster=w281, "Drive Encoder reset"=FALSE) -> (w282:T11)
                n194 = global write "Robot Values.vi" "Drive"(w282) -> ()
                n195 = Select(t=T4."Push", s=w286, f=T4."Start") -> (s? t:f=w287:T4)
                n196 = case shown="True" w286 {
                  frame False {
                  }
                  frame True {
                    n197 = local read "Totes grabed"() -> (w291:i32)
                    n198 = Increment(x=w291) -> (x+1=w290:i32)
                    n199 = local write "Totes grabed"(w290) -> ()
                  }
                }
              }
              frame "Nothing", Default {
                # "Do nothing, this should never be reached unless an error has occured.\nIf an error has occured, this case should activate and stop the robot\nto prevent failure."
              }
            }
          }
          "Total totes 2" <- 2 ("Total totes")
        }
        frame "1 Tote" {
          n200 = while {
            shift-right: [w300] -> _
            shift-left: T4."Start" -> [w301]
            tunnel: w294 -> [w298]
            tunnel: w293 -> [w297]
            stop <- FALSE stop-if-true
            n201 = case shown="\"Finish\"" w301 {
              tunnel: [w313 w328 w342 w352 w396 T4."Nothing"] -> w300
              tunnel: w298 -> [_ w324 _ _ _ _]
              tunnel: w297 -> [_ _ _ _ _ _]
              frame "Push" {
                # "chute door?"
                # "STILL NEED TO ADD TO WHEEL MOTORS TO PUSH IT OUT OF THE WAY!!\nMay need to delay starting the push case to check that no totes we are \ncarrying will interfere with pushing the green bin out of the way."
                # "Push green bin out of the way with wheels THEN move forward 206.74cm"
                n202 = global read "Robot Values.vi" "Tote Stopper Motors"() -> (w310:cluster{"RelayValue":T5, "RelayValue 2":T5})
                n203 = Bundle By Name(cluster=w310, "RelayValue"=WPI_RelayValue."Forward", "RelayValue 2"=WPI_RelayValue."Forward") -> (w311:cluster{"RelayValue":T5, "RelayValue 2":T5})
                n204 = global write "Robot Values.vi" "Tote Stopper Motors"(w311) -> ()
                n205 = global read "Robot Values.vi" "Drive"() -> (w305:T11)
                n206 = Unbundle By Name(w305) -> ("Right Wheel \n(Cm)"=w303:dbl)
                n207 = call "Auton go linear distance.vi"("PID setpoint"=130.0, "Goal"=130.0) -> ("Done?"=w307:bool)  [unwired: 6 in]
                n208 = Greater?(x=30.0, y=w303) -> (0:w302:bool)
                n209 = case shown="True" w302 {
                  frame False {
                  }
                  frame True {
                    n210 = global read "Robot Values.vi" "Tote Stopper Motors"() -> (w317:cluster{"RelayValue":T5, "RelayValue 2":T5})
                    n211 = Bundle By Name(cluster=w317, "RelayValue"=WPI_RelayValue."Reverse", "RelayValue 2"=WPI_RelayValue."Reverse") -> (w316:cluster{"RelayValue":T5, "RelayValue 2":T5})
                    n212 = global write "Robot Values.vi" "Tote Stopper Motors"(w316) -> ()
                  }
                }
                n213 = case shown="True" w307 {
                  frame False {
                  }
                  frame True {
                    n214 = global read "Robot Values.vi" "Drive"() -> (w321:T11)
                    n215 = Bundle By Name(cluster=w321, "Drive Encoder reset"=TRUE) -> (w322:T11)
                    n216 = global write "Robot Values.vi" "Drive"(w322) -> ()
                  }
                }
                n217 = Select(t=T4."Stack", s=w307, f=T4."Push") -> (s? t:f=w313:T4)
              }
              frame "Finish" {
                # "Russ did this"
                # "Drop arms while moving forward"
                # "Drive foraward 304.8 cm"
                n218 = global read "Robot Values.vi" "Drive"() -> (w330:T11)
                n219 = Bundle By Name(cluster=w330, "Drive Encoder reset"=FALSE) -> (w331:T11)
                n220 = global read "Robot Values.vi" "Lift System"() -> (w326:T12)
                n221 = Bundle By Name(cluster=w326, "Lift Position"=0) -> (w327:T12)
                n222 = global write "Robot Values.vi" "Lift System"(w327) -> ()
                n223 = global write "Robot Values.vi" "Drive"(w331) -> ()
                n224 = call "Auton go linear distance.vi"("Average gains"=w324, "PID setpoint"=452.0, "Goal"=450.0, "output range"=cluster{"output high":dbl, "output low":dbl} {"output high"=0.65, "output low"=-0.65}) -> ("Done?"=w332:bool)  [unwired: 4 in]
                n225 = case shown="True" w332 {
                  tunnel: [T4."Finish" T4."Nothing"] -> w328
                  frame False {
                  }
                  frame True {
                    # "Once finished expell the totes\nfrom the robot and that should\npush them out of the frame of\nthe robot so we are able to score\npoints for the stack."
                    n226 = global read "Robot Values.vi" "Tote Stopper Motors"() -> (w338:cluster{"RelayValue":T5, "RelayValue 2":T5})
                    n227 = Bundle By Name(cluster=w338, "RelayValue"=WPI_RelayValue."Forward", "RelayValue 2"=WPI_RelayValue."Forward") -> (w339:cluster{"RelayValue":T5, "RelayValue 2":T5})
                    n228 = global write "Robot Values.vi" "Tote Stopper Motors"(w339) -> ()
                  }
                }
              }
              frame "Turn" {
                # "HAVE TO ADJUST GAINS WHEN TESTING"
                # "Turn the robot 90 degres to the right"
                n229 = flat-sequence {
                  tunnel: [w348] -> w341
                  frame #0 {
                    n230 = global read "Robot Values.vi" "Sensors"() -> (w346:T13)
                    n231 = Bundle By Name(cluster=w346, "Gyro Reset"=FALSE) -> (w345:T13)
                    n232 = global write "Robot Values.vi" "Sensors"(w345) -> ()
                  }
                  frame #1 {
                    n233 = call "Auton Turn to disired angle.vi"("Power output range"="turn output range 3", "PID Turn  gains"="PID Turn  gains 3", "Angle setpoint"=90.0) -> ("In Range?"=w348:bool)  [unwired: 8 in]
                  }
                }
                n234 = Select(t=T4."Finish", s=w341, f=T4."Turn") -> (s? t:f=w342:T4)
              }
              frame "Stack" {
                # "Drop totes on top of new tote then pickup the new tote"
                n235 = flat-sequence {
                  tunnel: [w383] -> w352
                  frame #0 {
                    # "Note: Time value might \nneed to be adjusted"
                    n236 = global read "Robot Values.vi" "Tote Stopper Motors"() -> (w355:cluster{"RelayValue":T5, "RelayValue 2":T5})
                    n237 = Bundle By Name(cluster=w355, "RelayValue"=WPI_RelayValue."Off", "RelayValue 2"=WPI_RelayValue."Off") -> (w356:cluster{"RelayValue":T5, "RelayValue 2":T5})
                    n238 = global read "Robot Values.vi" "Lift System"() -> (w359:T12)
                    n239 = Bundle By Name(cluster=w359, "Lift Position"=0) -> (w358:T12)
                    n240 = global write "Robot Values.vi" "Tote Stopper Motors"(w356) -> ()
                    n241 = Wait (ms)(milliseconds to wait=u32 1200) -> ()  [unwired: 1 out]
                    n242 = global write "Robot Values.vi" "Lift System"(w358) -> ()
                  }
                  frame #1 {
                    # "100 delay becuase we want to try to lift\nthe tote and move onto the next case"
                    n243 = local read "Total totes 3"() -> (w363:i32)
                    n244 = local read "Totes grabed"() -> (w362:i32)
                    n245 = Decrement(x=w362) -> (x-1=w361:i32)
                    n246 = Equal?(x=w363, y=w361) -> (x = y?=w367:bool)
                    n247 = Select(t=0 ("Lift Position"), s=w367, f=2 ("Lift Position")) -> (s? t:f=w364:i32)
                    n248 = Wait (ms)(milliseconds to wait=u32 100) -> ()  [unwired: 1 out]
                    n249 = global read "Robot Values.vi" "Lift System"() -> (w369:T12)
                    n250 = Bundle By Name(cluster=w369, "Lift Position"=w364) -> (w370:T12)
                    n251 = global write "Robot Values.vi" "Lift System"(w370) -> ()
                  }
                  frame #2 {
                    n252 = global read "Robot Values.vi" "Drive"() -> (w374:T11)
                    n253 = Bundle By Name(cluster=w374, "Drive Encoder reset"=FALSE) -> (w375:T11)
                    n254 = local read "Totes grabed"() -> (w371:i32)
                    n255 = local read "Total totes 3"() -> (w382:i32)
                    n256 = global read "Robot Values.vi" "Sensors"() -> (w377:T13)
                    n257 = global write "Robot Values.vi" "Drive"(w375) -> ()
                    n258 = Bundle By Name(cluster=w377, "Gyro Reset"=TRUE) -> (w378:T13)
                    n259 = Increment(x=w371) -> (x+1=w372:i32)
                    n260 = Equal?(x=w371, y=w382) -> (x = y?=w380:bool)
                    n261 = global write "Robot Values.vi" "Sensors"(w378) -> ()
                    n262 = local write "Totes grabed"(w372) -> ()
                    n263 = Select(t=T4."Turn", s=w380, f=T4."Push") -> (s? t:f=w383:T4)
                  }
                }
              }
              frame "Start" {
                w395 = TRUE  # Is finished
                # "Selector is left in case testing fails\nand it needs to switch."
                # "Will switch to push state after starting to\nlift the tote."
                # "Is finished is set to true because\nthe robot will lift the tote while\nit is moving forawrd in the\n\"Push\" state.\n\nThis still needs to be tested.\nAnother possible solution is a\ntimed delay if simoultaneous\ntesting fails."
                # "Grab and then lift first tote"
                n264 = global read "Robot Values.vi" "Lift System"() -> (w393:T12)
                n265 = Bundle By Name(cluster=w393, "Lift Position"=0) -> (w394:T12)
                n266 = global write "Robot Values.vi" "Lift System"(w394) -> ()
                n267 = global read "Robot Values.vi" "Tote Stopper Motors"() -> (w386:cluster{"RelayValue":T5, "RelayValue 2":T5})
                n268 = Bundle By Name(cluster=w386, "RelayValue"=WPI_RelayValue."Off", "RelayValue 2"=WPI_RelayValue."Off") -> (w387:cluster{"RelayValue":T5, "RelayValue 2":T5})
                n269 = global write "Robot Values.vi" "Tote Stopper Motors"(w387) -> ()
                n270 = Wait (ms)(milliseconds to wait=u32 50) -> ()  [unwired: 1 out]
                n271 = global read "Robot Values.vi" "Drive"() -> (w390:T11)
                n272 = Bundle By Name(cluster=w390, "Drive Encoder reset"=FALSE) -> (w391:T11)
                n273 = global write "Robot Values.vi" "Drive"(w391) -> ()
                n274 = Select(t=T4."Turn", s=w395, f=T4."Start") -> (s? t:f=w396:T4)
                n275 = case shown="True" w395 {
                  frame False {
                  }
                  frame True {
                    n276 = local read "Totes grabed"() -> (w400:i32)
                    n277 = Increment(x=w400) -> (x+1=w399:i32)
                    n278 = local write "Totes grabed"(w399) -> ()
                  }
                }
              }
              frame "Nothing", Default {
                w401 = 0.0
                # "Do nothing, this should never be reached unless an error has occured.\nIf an error has occured, this case should activate and stop the robot\nto prevent failure."
                n279 = global read "DriveGlobal.vi" "Drive speeds"() -> (w402:T10)
                n280 = Bundle By Name(cluster=w402, "RightMotorSpeed"=w401, "LeftMotorSpeed"=w401) -> (w403:T10)
                n281 = global write "DriveGlobal.vi" "Drive speeds"(w403) -> ()
              }
            }
          }
          "Total totes 3" <- 0 ("Total totes")
        }
        frame "Blank 1" {
          n282 = disable-structure shown="Disabled" {
            frame Disabled {
              n283 = global read "Robot Values.vi" "Lift System"() -> (w427:T12)
              n284 = Bundle By Name(cluster=w427, "Lift Position"=2) -> (w428:T12)
              n285 = global read "Robot Values.vi" "Tote Stopper Motors"() -> (w424:cluster{"RelayValue":T5, "RelayValue 2":T5})
              n286 = Bundle By Name(cluster=w424, "RelayValue"=WPI_RelayValue."Off", "RelayValue 2"=WPI_RelayValue."Off") -> (w425:cluster{"RelayValue":T5, "RelayValue 2":T5})
              n287 = global write "Robot Values.vi" "Lift System"(w428) -> ()
              n288 = global write "Robot Values.vi" "Tote Stopper Motors"(w425) -> ()
            }
            frame Enabled {
            }
          }
          n289 = flat-sequence {
            tunnel: w405 -> [w406]
            frame #0 {
              n290 = while {
                tunnel: w406 -> [w417]
                tunnel: cluster{"output high":dbl, "output low":dbl} {"output high"=0.5, "output low"=-0.5} ("output range") -> [w416]
                stop <- w409 stop-if-true
                n291 = global read "Robot Values.vi" "Auton"() -> (w412:cluster{"Auton":string, "Pushing tote":bool})
                n292 = Unbundle By Name(w412) -> ("Pushing tote"=w411:bool)
                n293 = Select(t=600.0, s=w411, f=400.0 ("PID setpoint")) -> (s? t:f=w414:dbl)
                n294 = call "Auton go linear distance.vi"("Average gains"=w417, "PID setpoint"=w414, "Goal"=w414, "output range"=w416) -> ("Done?"=w410:bool)  [unwired: 4 in]
                n295 = call "Elapsed Time2"() -> ("Time has Elapsed"=w408:bool)  [unwired: 12 in, 7 out]
                n296 = Or(x=w408, y=w410) -> (x .or. y?=w409:bool)
              }
            }
            frame #1 {
              n297 = global read "DriveGlobal.vi" "Drive speeds"() -> (w420:T10)
              n298 = Bundle By Name(cluster=w420, "RightMotorSpeed"=0.0, "LeftMotorSpeed"=0.0) -> (w421:T10)
              n299 = global write "DriveGlobal.vi" "Drive speeds"(w421) -> ()
            }
          }
        }
        frame "Blank 2" {
          n300 = while {
            shift-right: [w436] -> _
            shift-left: AutonEnum."Start" -> [w437]
            tunnel: w430 -> [w434]
            tunnel: w431 -> [w433]
            stop <- FALSE stop-if-true
            n301 = case shown="\"Turn\"" w437 {
              tunnel: [w453 w464 w482 w496 w621 w647 AutonEnum."Nothing" w682 AutonEnum."Nothing"] -> w436
              tunnel: w434 -> [w451 w469 _ w501 _ w651 _ _ _]
              tunnel: w433 -> [w452 w470 _ w502 _ w650 _ _ _]
              frame "Push" {
                # "chute door?"
                # "STILL NEED TO ADD TO WHEEL MOTORS TO PUSH IT OUT OF THE WAY!!\nMay need to delay starting the push case to check that no totes we are \ncarrying will interfere with pushing the green bin out of the way."
                # "Push green bin out of the way with wheels THEN move forward 206.74cm"
                n302 = global read "Robot Values.vi" "Tote Stopper Motors"() -> (w448:cluster{"RelayValue":T5, "RelayValue 2":T5})
                n303 = Bundle By Name(cluster=w448, "RelayValue"=WPI_RelayValue."Forward", "RelayValue 2"=WPI_RelayValue."Forward") -> (w449:cluster{"RelayValue":T5, "RelayValue 2":T5})
                n304 = global write "Robot Values.vi" "Tote Stopper Motors"(w449) -> ()
                n305 = global read "Robot Values.vi" "Drive"() -> (w443:T11)
                n306 = Unbundle By Name(w443) -> ("Right Wheel \n(Cm)"=w441:dbl)
                n307 = call "Auton go linear distance.vi"("Average gains"=w451, "PID setpoint"=130.0, "Goal"=130.0, "output range"=w452) -> ("Done?"=w445:bool)  [unwired: 4 in]
                n308 = Greater?(x=30.0, y=w441) -> (0:w440:bool)
                n309 = case shown="True" w440 {
                  frame False {
                  }
                  frame True {
                    n310 = global read "Robot Values.vi" "Tote Stopper Motors"() -> (w455:cluster{"RelayValue":T5, "RelayValue 2":T5})
                    n311 = Bundle By Name(cluster=w455, "RelayValue"=WPI_RelayValue."Reverse", "RelayValue 2"=WPI_RelayValue."Reverse") -> (w454:cluster{"RelayValue":T5, "RelayValue 2":T5})
                    n312 = global write "Robot Values.vi" "Tote Stopper Motors"(w454) -> ()
                  }
                }
                n313 = case shown="True" w445 {
                  frame False {
                  }
                  frame True {
                    n314 = global read "Robot Values.vi" "Drive"() -> (w459:T11)
                    n315 = Bundle By Name(cluster=w459, "Drive Encoder reset"=TRUE) -> (w460:T11)
                    n316 = global write "Robot Values.vi" "Drive"(w460) -> ()
                  }
                }
                n317 = Select(t=AutonEnum."Stack", s=w445, f=AutonEnum."Push") -> (s? t:f=w453:T7)
              }
              frame "Finish" {
                # "Drop arms while moving forward"
                # "Drive foraward 304.8 cm"
                n318 = global read "Robot Values.vi" "Drive"() -> (w466:T11)
                n319 = Bundle By Name(cluster=w466, "Drive Encoder reset"=FALSE) -> (w467:T11)
                n320 = global read "Robot Values.vi" "Lift System"() -> (w462:T12)
                n321 = Bundle By Name(cluster=w462, "Lift Position"=0) -> (w463:T12)
                n322 = global write "Robot Values.vi" "Lift System"(w463) -> ()
                n323 = global write "Robot Values.vi" "Drive"(w467) -> ()
                n324 = call "Auton go linear distance.vi"("Average gains"=w469, "PID setpoint"=70.0, "Goal"=70.0, "output range"=w470) -> ("Done?"=w468:bool)  [unwired: 4 in]
                n325 = case shown="True" w468 {
                  tunnel: [AutonEnum."Finish" AutonEnum."Finish"] -> w464
                  frame False {
                  }
                  frame True {
                    # "Once finished expell the totes\nfrom the robot and that should\npush them out of the frame of\nthe robot so we are able to score\npoints for the stack."
                    n326 = global read "Robot Values.vi" "Tote Stopper Motors"() -> (w477:cluster{"RelayValue":T5, "RelayValue 2":T5})
                    n327 = Bundle By Name(cluster=w477, "RelayValue"=WPI_RelayValue."Forward", "RelayValue 2"=WPI_RelayValue."Forward") -> (w478:cluster{"RelayValue":T5, "RelayValue 2":T5})
                    n328 = global write "Robot Values.vi" "Tote Stopper Motors"(w478) -> ()
                  }
                }
              }
              frame "Turn" {
                # "HAVE TO ADJUST GAINS WHEN TESTING"
                # "Turn the robot 90 degres to the right"
                n329 = flat-sequence {
                  tunnel: [w486] -> w481
                  frame #0 {
                    n330 = global read "Robot Values.vi" "Sensors"() -> (w484:T13)
                    n331 = Bundle By Name(cluster=w484, "Gyro Reset"=FALSE) -> (w483:T13)
                    n332 = global write "Robot Values.vi" "Sensors"(w483) -> ()
                  }
                  frame #1 {
                    n333 = call "Auton Turn to disired angle.vi"("Power output range"="turn output range 4", "PID Turn  gains"="PID Turn  gains 4", "Angle setpoint"=45.0) -> ("In Range?"=w486:bool)  [unwired: 8 in]
                    n334 = case shown="True" w486 {
                      frame False {
                      }
                      frame True {
                        n335 = Wait (ms)(milliseconds to wait=u32 20) -> ()  [unwired: 1 out]
                        n336 = global read "Robot Values.vi" "Drive"() -> (w492:T11)
                        n337 = Bundle By Name(cluster=w492, "Drive Encoder reset"=TRUE) -> (w493:T11)
                        n338 = global write "Robot Values.vi" "Drive"(w493) -> ()
                      }
                    }
                  }
                }
                n339 = Select(t=AutonEnum."To Auto", s=w481, f=AutonEnum."Turn") -> (s? t:f=w482:T7)
              }
              frame "Go Around" {
                n340 = while {
                  shift-right: [w508] -> _
                  shift-left: AutonEnumGoAround."Turn Right 1" -> [w509]
                  tunnel: w502 -> [w507]
                  tunnel: w501 -> [w506]
                  tunnel: [w505] -> w499
                  tunnel: "turn output range 5" -> [w504]
                  tunnel: "PID Turn  gains 5" -> [w503]
                  stop <- w505 stop-if-true
                  n341 = case shown="\"Turn Left 2\"" w509 {
                    tunnel: [w515 w529 w540 w551 w565 w586 w597 w613 AutonEnumGoAround."Nothing"] -> w508
                    tunnel: w507 -> [_ w531 _ w552 _ _ _ w614 _]
                    tunnel: w506 -> [_ w530 _ w553 _ w587 _ w615 _]
                    tunnel: [FALSE FALSE FALSE FALSE FALSE FALSE FALSE FALSE TRUE] -> w505
                    tunnel: w504 -> [w512 _ w536 _ w563 _ w594 _ _]
                    tunnel: w503 -> [w511 _ w535 _ w562 _ w593 _ _]
                    frame "Turn Right 1" {
                      n342 = call "Auton Turn to disired angle.vi"("Power output range"=w512, "PID Turn  gains"=w511, "Angle setpoint"=35.0) -> ("In Range?"=w510:bool)  [unwired: 8 in]
                      n343 = Select(t=AutonEnumGoAround."Go Straight 1", s=w510, f=AutonEnumGoAround."Turn Right 1") -> (s? t:f=w515:T8)
                      n344 = case shown="True" w510 {
                        frame False {
                        }
                        frame True {
                          n345 = global read "Robot Values.vi" "Drive"() -> (w520:T11)
                          n346 = Bundle By Name(cluster=w520, "Drive Encoder reset"=TRUE) -> (w521:T11)
                          n347 = global write "Robot Values.vi" "Drive"(w521) -> ()
                          n348 = Wait (ms)(milliseconds to wait=u32 20) -> ()  [unwired: 1 out]
                        }
                      }
                    }
                    frame "Go Straight 1" {
                      n349 = call "Auton go linear distance.vi"("Average gains"=w530, "PID setpoint"=50.0, "Goal"=50.0, "output range"=w531) -> ("Done?"=w525:bool)  [unwired: 4 in]
                      n350 = Select(t=AutonEnumGoAround."Turn Left 1", s=w525, f=AutonEnumGoAround."Go Straight 1") -> (s? t:f=w529:T8)
                      n351 = global read "Robot Values.vi" "Drive"() -> (w523:T11)
                      n352 = Bundle By Name(cluster=w523, "Drive Encoder reset"=FALSE) -> (w524:T11)
                      n353 = global write "Robot Values.vi" "Drive"(w524) -> ()
                    }
                    frame "Turn Left 1" {
                      n354 = call "Auton Turn to disired angle.vi"("Power output range"=w536, "PID Turn  gains"=w535, "Angle setpoint"=-40.0) -> ("In Range?"=w534:bool)  [unwired: 8 in]
                      n355 = Select(t=AutonEnumGoAround."Go Straight 2", s=w534, f=AutonEnumGoAround."Turn Left 1") -> (s? t:f=w540:T8)
                      n356 = case shown="True" w534 {
                        frame False {
                        }
                        frame True {
                          n357 = global read "Robot Values.vi" "Drive"() -> (w544:T11)
                          n358 = Bundle By Name(cluster=w544, "Drive Encoder reset"=TRUE) -> (w545:T11)
                          n359 = global write "Robot Values.vi" "Drive"(w545) -> ()
                          n360 = Wait (ms)(milliseconds to wait=u32 20) -> ()  [unwired: 1 out]
                        }
                      }
                    }
                    frame "Go Straight 2" {
                      n361 = call "Auton go linear distance.vi"("Average gains"=w553, "PID setpoint"=81.0, "Goal"=78.0, "output range"=w552) -> ("Done?"=w549:bool)  [unwired: 4 in]
                      n362 = Select(t=AutonEnumGoAround."Turn Left 2", s=w549, f=AutonEnumGoAround."Go Straight 2") -> (s? t:f=w551:T8)
                      n363 = global read "Robot Values.vi" "Drive"() -> (w548:T11)
                      n364 = Bundle By Name(cluster=w548, "Drive Encoder reset"=FALSE) -> (w547:T11)
                      n365 = global write "Robot Values.vi" "Drive"(w547) -> ()
                    }
                    frame "Turn Left 2" {
                      # "Now a turn right"
                      n366 = global read "Robot Values.vi" "Lift System"() -> (w559:T12)
                      n367 = Bundle By Name(cluster=w559, "Lift Position"=2) -> (w560:T12)
                      n368 = global write "Robot Values.vi" "Lift System"(w560) -> ()
                      n369 = call "Auton Turn to disired angle.vi"("Power output range"=w563, "PID Turn  gains"=w562, "Angle setpoint"=-6.0) -> ("In Range?"=w561:bool)  [unwired: 8 in]
                      n370 = Select(t=AutonEnumGoAround."Go Straight 3", s=w561, f=AutonEnumGoAround."Turn Left 2") -> (s? t:f=w565:T8)
                      n371 = case shown="True" w561 {
                        frame False {
                        }
                        frame True {
                          n372 = global read "Robot Values.vi" "Drive"() -> (w572:T11)
                          n373 = Bundle By Name(cluster=w572, "Drive Encoder reset"=TRUE) -> (w571:T11)
                          n374 = global write "Robot Values.vi" "Drive"(w571) -> ()
                          n375 = Wait (ms)(milliseconds to wait=u32 20) -> ()  [unwired: 1 out]
                        }
                      }
                    }
                    frame "Go Straight 3" {
                      n376 = call "Auton go linear distance.vi"("Average gains"=w587, "PID setpoint"=77.0, "Goal"=77.0, "output range"=cluster{"output high":dbl, "output low":dbl} {"output high"=0.5, "output low"=-0.5}) -> ("Done?"=w584:bool)  [unwired: 4 in]
                      n377 = Select(t=AutonEnumGoAround."Nothing", s=w584, f=AutonEnumGoAround."Go Straight 3") -> (s? t:f=w586:T8)
                      n378 = global read "Robot Values.vi" "Lift System"() -> (w579:T12)
                      n379 = Bundle By Name(cluster=w579, "Lift Position"=2) -> (w580:T12)
                      n380 = global read "Robot Values.vi" "Tote Stopper Motors"() -> (w577:cluster{"RelayValue":T5, "RelayValue 2":T5})
                      n381 = Bundle By Name(cluster=w577, "RelayValue"=WPI_RelayValue."Reverse", "RelayValue 2"=WPI_RelayValue."Forward") -> (w574:cluster{"RelayValue":T5, "RelayValue 2":T5})
                      n382 = global write "Robot Values.vi" "Lift System"(w580) -> ()
                      n383 = global read "Robot Values.vi" "Drive"() -> (w582:T11)
                      n384 = Bundle By Name(cluster=w582, "Drive Encoder reset"=FALSE) -> (w583:T11)
                      n385 = global write "Robot Values.vi" "Tote Stopper Motors"(w574) -> ()
                      n386 = global write "Robot Values.vi" "Drive"(w583) -> ()
                    }
                    frame "Turn Right 3" {
                      # "Not in use"
                      n387 = call "Auton Turn to disired angle.vi"("Power output range"=w594, "PID Turn  gains"=w593, "Angle setpoint"=0.0) -> ("In Range?"=w592:bool)  [unwired: 8 in]
                      n388 = Select(t=AutonEnumGoAround."Go Straight 4", s=w592, f=AutonEnumGoAround."Turn Right 3") -> (s? t:f=w597:T8)
                      n389 = case shown="True" w592 {
                        frame False {
                        }
                        frame True {
                          n390 = global read "Robot Values.vi" "Drive"() -> (w602:T11)
                          n391 = Bundle By Name(cluster=w602, "Drive Encoder reset"=TRUE) -> (w603:T11)
                          n392 = global write "Robot Values.vi" "Drive"(w603) -> ()
                          n393 = Wait (ms)(milliseconds to wait=u32 20) -> ()  [unwired: 1 out]
                        }
                      }
                    }
                    frame "Go Straight 4" {
                      # "Not in use"
                      n394 = call "Auton go linear distance.vi"("Average gains"=w615, "PID setpoint"=30.0, "Goal"=30.0, "output range"=w614) -> ("Done?"=w608:bool)  [unwired: 4 in]
                      n395 = Select(t=AutonEnumGoAround."Nothing", s=w608, f=AutonEnumGoAround."Go Straight 4") -> (s? t:f=w613:T8)
                      n396 = global read "Robot Values.vi" "Lift System"() -> (w605:T12)
                      n397 = Bundle By Name(cluster=w605, "Lift Position"=2) -> (w604:T12)
                      n398 = global write "Robot Values.vi" "Lift System"(w604) -> ()
                      n399 = global read "Robot Values.vi" "Drive"() -> (w609:T11)
                      n400 = Bundle By Name(cluster=w609, "Drive Encoder reset"=FALSE) -> (w610:T11)
                      n401 = global write "Robot Values.vi" "Drive"(w610) -> ()
                    }
                    frame "Nothing", Default {
                    }
                  }
                }
                n402 = Select(t=AutonEnum."Stack", s=w499, f=AutonEnum."Go Around") -> (s? t:f=w496:T7)
              }
              frame "Stack" {
                # "Drop totes on top of new tote then pickup the new tote"
                n403 = flat-sequence {
                  tunnel: [w631] -> w621
                  frame #0 {
                    n404 = Wait (ms)(milliseconds to wait=u32 250) -> ()  [unwired: 1 out]
                  }
                  frame #1 {
                    # "Note: Time value might \nneed to be adjusted"
                    n405 = global read "Robot Values.vi" "Tote Stopper Motors"() -> (w625:cluster{"RelayValue":T5, "RelayValue 2":T5})
                    n406 = Bundle By Name(cluster=w625, "RelayValue"=WPI_RelayValue."Off", "RelayValue 2"=WPI_RelayValue."Off") -> (w626:cluster{"RelayValue":T5, "RelayValue 2":T5})
                    n407 = global read "Robot Values.vi" "Lift System"() -> (w629:T12)
                    n408 = Bundle By Name(cluster=w629, "Lift Position"=0) -> (w628:T12)
                    n409 = global write "Robot Values.vi" "Tote Stopper Motors"(w626) -> ()
                    n410 = Wait (ms)(milliseconds to wait=u32 1000) -> ()  [unwired: 1 out]
                    n411 = global write "Robot Values.vi" "Lift System"(w628) -> ()
                  }
                  frame #2 {
                    n412 = global read "Robot Values.vi" "Drive"() -> (w637:T11)
                    n413 = Bundle By Name(cluster=w637, "Drive Encoder reset"=FALSE) -> (w638:T11)
                    n414 = local read "Totes grabed"() -> (w635:i32)
                    n415 = local read "Total totes 4"() -> (w643:i32)
                    n416 = global read "Robot Values.vi" "Sensors"() -> (w640:T13)
                    n417 = global write "Robot Values.vi" "Drive"(w638) -> ()
                    n418 = Bundle By Name(cluster=w640, "Gyro Reset"=TRUE) -> (w641:T13)
                    n419 = Increment(x=w635) -> (x+1=w634:i32)
                    n420 = global write "Robot Values.vi" "Sensors"(w641) -> ()
                    n421 = local write "Totes grabed"(w634) -> ()
                    n422 = Equal?(x=w635, y=w643) -> (x = y?=w642:bool)
                    n423 = Select(t=AutonEnum."Turn", s=w642, f=AutonEnum."Go Around") -> (s? t:f=w631:T7)
                  }
                }
              }
              frame "To Auto" {
                n424 = call "Auton go linear distance.vi"("Average gains"=w651, "PID setpoint"=300.0, "Goal"=300.0 ("Max"), "output range"=w650) -> ("Done?"=w646:bool)  [unwired: 4 in]
                n425 = case shown="True" w646 {
                  frame False {
                  }
                  frame True {
                    n426 = global read "Robot Values.vi" "Drive"() -> (w653:T11)
                    n427 = Bundle By Name(cluster=w653, "Drive Encoder reset"=TRUE) -> (w655:T11)
                    n428 = global write "Robot Values.vi" "Drive"(w655) -> ()
                    n429 = Wait (ms)(milliseconds to wait=u32 20) -> ()  [unwired: 1 out]
                  }
                }
                n430 = Select(t=AutonEnum."Release Totes", s=w646, f=AutonEnum."To Auto") -> (s? t:f=w647:T7)
              }
              frame "Release Totes" {
                w656 = -0.4
                n431 = global read "Robot Values.vi" "Tote Stopper Motors"() -> (w663:cluster{"RelayValue":T5, "RelayValue 2":T5})
                n432 = Bundle By Name(cluster=w663, "RelayValue"=WPI_RelayValue."Forward", "RelayValue 2"=WPI_RelayValue."Reverse") -> (w660:cluster{"RelayValue":T5, "RelayValue 2":T5})
                n433 = global write "Robot Values.vi" "Tote Stopper Motors"(w660) -> ()
                n434 = global read "DriveGlobal.vi" "Drive speeds"() -> (w657:T10)
                n435 = Bundle By Name(cluster=w657, "RightMotorSpeed"=w656, "LeftMotorSpeed"=w656) -> (w658:T10)
                n436 = global write "DriveGlobal.vi" "Drive speeds"(w658) -> ()
                n437 = Wait (ms)(milliseconds to wait=u32 1000) -> ()  [unwired: 1 out]
              }
              frame "Start" {
                w681 = TRUE  # Is finished
                # "Selector is left in case testing fails\nand it needs to switch."
                # "Will switch to push state after starting to\nlift the tote."
                # "Is finished is set to true because\nthe robot will lift the tote while\nit is moving forawrd in the\n\"Push\" state.\n\nThis still needs to be tested.\nAnother possible solution is a\ntimed delay if simoultaneous\ntesting fails."
                # "Grab and then lift first tote"
                n438 = global read "Robot Values.vi" "Tote Stopper Motors"() -> (w668:cluster{"RelayValue":T5, "RelayValue 2":T5})
                n439 = Bundle By Name(cluster=w668, "RelayValue"=WPI_RelayValue."Off", "RelayValue 2"=WPI_RelayValue."Off") -> (w665:cluster{"RelayValue":T5, "RelayValue 2":T5})
                n440 = global write "Robot Values.vi" "Tote Stopper Motors"(w665) -> ()
                n441 = global read "Robot Values.vi" "Sensors"() -> (w673:T13)
                n442 = Bundle By Name(cluster=w673, "Gyro Reset"=FALSE) -> (w674:T13)
                n443 = global write "Robot Values.vi" "Sensors"(w674) -> ()
                n444 = Wait (ms)(milliseconds to wait=u32 50) -> ()  [unwired: 1 out]
                n445 = global read "Robot Values.vi" "Drive"() -> (w679:T11)
                n446 = Bundle By Name(cluster=w679, "Drive Encoder reset"=FALSE) -> (w680:T11)
                n447 = global write "Robot Values.vi" "Drive"(w680) -> ()
                n448 = Select(t=AutonEnum."Go Around", s=w681, f=AutonEnum."Start") -> (s? t:f=w682:T7)
                n449 = global read "Robot Values.vi" "Lift System"() -> (w670:T12)
                n450 = Bundle By Name(cluster=w670, "Lift Position"=0) -> (w669:T12)
                n451 = case shown="True" w681 {
                  frame False {
                  }
                  frame True {
                    n452 = local read "Totes grabed"() -> (w684:i32)
                    n453 = Increment(x=w684) -> (x+1=w683:i32)
                    n454 = local write "Totes grabed"(w683) -> ()
                  }
                }
                n455 = global write "Robot Values.vi" "Lift System"(w669) -> ()
              }
              frame "Nothing", Default {
                # "Do nothing, this should never be reached unless an error has occured.\nIf an error has occured, this case should activate and stop the robot\nto prevent failure."
              }
            }
          }
          "Total totes 4" <- 1 ("Total totes")
        }
      }
      "Totes grabed" <- 0 ("Totes grabed")
    }
    frame Disabled {
      n456 = while {
        shift-right: [w688] -> _
        shift-left: Auton1ToteEnum."First Forward" -> [w689]
        stop <- FALSE stop-if-true
        n457 = case shown="\"First Forward\"" w689 {
          selector: w689 -> [_ _ _ w712 w717]
          tunnel: [Auton1ToteEnum."First Forward" w702 Auton1ToteEnum."First Pick Up" w712 w717] -> w688
          frame "Start", Default {
            n458 = global read "Robot Values.vi" "Lift System"() -> (w694:T12)
            n459 = Bundle By Name(cluster=w694, "Lift Position"=2) -> (w693:T12)
            n460 = global write "Robot Values.vi" "Lift System"(w693) -> ()
            n461 = Wait (ms)(milliseconds to wait=u32 5000) -> ()  [unwired: 1 out]
          }
          frame "First Forward" {
            n462 = call "Auton go linear distance.vi"("Average gains"="Average gains", "PID setpoint"=254.0 ("setpoint"), "Goal"=254.0 ("y"), "output range"=cluster{"output high":dbl, "output low":dbl} {"output high"=0.35, "output low"=-0.35}) -> ("Done?"=w695:bool)  [unwired: 4 in]
            n463 = Select(t=Auton1ToteEnum."Get First Tote", s=w695, f=Auton1ToteEnum."First Forward") -> (s? t:f=w702:T9)
          }
          frame "Get First Tote" {
            n464 = global read "Robot Values.vi" "Lift System"() -> (w711:T12)
            n465 = Bundle By Name(cluster=w711, "Lift Position"=0) -> (w710:T12)
            n466 = global write "Robot Values.vi" "Lift System"(w710) -> ()
            n467 = global read "DriveGlobal.vi" "Drive speeds"() -> (w708:T10)
            n468 = Bundle By Name(cluster=w708, "RightMotorSpeed"=0.0, "LeftMotorSpeed"=0.0) -> (w707:T10)
            n469 = global write "DriveGlobal.vi" "Drive speeds"(w707) -> ()
            n470 = Wait (ms)(milliseconds to wait=u32 50) -> ()  [unwired: 1 out]
          }
          frame "First Pick Up" {
            n471 = global read "Robot Values.vi" "Lift System"() -> (w715:T12)
            n472 = Bundle By Name(cluster=w715, "Lift Position"=1) -> (w714:T12)
            n473 = global write "Robot Values.vi" "Lift System"(w714) -> ()
            n474 = Wait (ms)(milliseconds to wait=u32 50) -> ()  [unwired: 1 out]
          }
          frame "Stop" {
          }
        }
      }
    }
  }
  n475 = while {
    stop <- FALSE stop-if-true
    n476 = call <vilib>:"WPI_DriverStationReport Robot Code State.vi"("Autonomous"=TRUE) -> ()  [unwired: 10 in, 1 out]
    n477 = Wait (ms)(milliseconds to wait=u32 20) -> ()  [unwired: 1 out]
  }
  n478 = call <vilib>:"WPI_DriverStationGet Alliance Info.vi"() -> ()  [unwired: 12 out]
  n479 = call <vilib>:"WPI_JoystickRefNum Registry Get.vi"("refnum name"="Joystick 0") -> ("JoystickDevRef"=w3:T14)  [unwired: 1 in, 9 out]
  n480 = call <vilib>:"WPI_JoystickGetValues.vi"("JoystickDevRef"=w3) -> ("Axes"=w1:dbl[])  [unwired: 6 in, 4 out]
  n481 = call <vilib>:"SD Write Numeric Array.vi"("Numeric Array"=w1, "Name"="Joystick 0/Axes") -> ()  [unwired: 8 in, 2 out]
  n482 = disable-structure shown="Disabled" {
    frame Disabled {
      w724 = "RobotDrive Motors" ("Name")
      # "This is some simple sample code to drive your robot curving one direction and then the other."
      # "stand still"
      # "turn left for 0.5 second"
      # "turn right for 1 second"
      n483 = call <vilib>:"WPI_RobotDriveRefNum Registry Get.vi"("refnum name"="Left and Right Motors") -> ("RobotDriveDevRef"=w725:T16)  [unwired: 1 in, 9 out]
      n484 = call-poly <vilib>:"WPI_RobotDriveArcadeDrive.vi"("Y axis value"=0.5 ("X axis value"), "X axis value"=0.25, "RobotDriveDevRef"=w725) -> ("Motor Values"=w723:dbl[], "RobotDriveDevRef"=w732:T16)  [unwired: 1 in, 6 out]
      n485 = call-poly <vilib>:"SD Write Value.vi"("Numeric Array"=w723, "Name"=w724) -> ()  [unwired: 8 in, 2 out]
      n486 = call <vilib>:"WPI_RobotDriveDelayAndUpdateSafety.vi"("Delay (s)"=1.0, "RobotDriveDevRef"=w732) -> ("RobotDriveDevRef 2"=w731:T16)  [unwired: 8 in, 1 out]
      n487 = call-poly <vilib>:"WPI_RobotDriveArcadeDrive.vi"("Y axis value"=0.25 ("X axis value"), "X axis value"=0.5, "RobotDriveDevRef"=w731) -> ("Motor Values"=w722:dbl[], "RobotDriveDevRef"=w730:T16)  [unwired: 1 in, 6 out]
      n488 = call-poly <vilib>:"SD Write Value.vi"("Numeric Array"=w722, "Name"=w724) -> ()  [unwired: 8 in, 2 out]
      n489 = call <vilib>:"WPI_RobotDriveDelayAndUpdateSafety.vi"("Delay (s)"=0.5, "RobotDriveDevRef"=w730) -> ("RobotDriveDevRef 2"=w729:T16)  [unwired: 8 in, 1 out]
      n490 = call-poly <vilib>:"WPI_RobotDriveArcadeDrive.vi"("Y axis value"=0.0 ("X axis value"), "X axis value"=0.0, "RobotDriveDevRef"=w729) -> ("Motor Values"=w721:dbl[])  [unwired: 1 in, 7 out]
      n491 = call-poly <vilib>:"SD Write Value.vi"("Numeric Array"=w721, "Name"=w724) -> ()  [unwired: 8 in, 2 out]
    }
    frame Enabled {
    }
  }
  n492 = disable-structure shown="Disabled" {
    frame Disabled {
      # "This sample code describes robot movements in an array. You can extend it to control other motors\non your robot. You can also use file I/O to move the data to a text file."
      n493 = call <vilib>:"WPI_RobotDriveRefNum Registry Get.vi"("refnum name"="Left and Right Motors") -> ("RobotDriveDevRef"=w740:T16)  [unwired: 1 in, 9 out]
      n494 = for {
        shift-right: [w747] -> _
        shift-left: w740 -> [w748]
        tunnel: "Array of robot movements" -> [w743] mode=indexing
        n495 = Unbundle By Name(w743) -> ("X Joystick Value"=w746:dbl, "Y Joystick Value"=w745:dbl, "Delay (sec)"=w744:dbl)  [unwired: 1 out]
        n496 = call-poly <vilib>:"WPI_RobotDriveArcadeDrive.vi"("Y axis value"=w745, "X axis value"=w746, "RobotDriveDevRef"=w748) -> ("Motor Values"=w742:dbl[], "RobotDriveDevRef"=w749:T16)  [unwired: 1 in, 6 out]
        n497 = call-poly <vilib>:"SD Write Value.vi"("Numeric Array"=w742, "Name"="RobotDrive Motors") -> ()  [unwired: 8 in, 2 out]
        n498 = call <vilib>:"WPI_RobotDriveDelayAndUpdateSafety.vi"("Delay (s)"=w744, "RobotDriveDevRef"=w749) -> ("RobotDriveDevRef 2"=w747:T16)  [unwired: 8 in, 1 out]
        "Current Movement, for debugging" <- w743
      }
    }
    frame Enabled {
    }
  }
  n499 = Default Directory() -> ()  [unwired: 1 out]
